vi "MAIN.vi"() -> ()   [LabVIEW 2015]
doc: "Use this template to create an application that executes repeatedly until you click the Stop button. This template polls the state of the Stop button and does not use events. Use the Top-Level Application template (not available in the Base package) to create a single-loop application with event handling."
uses:
  <vilib>/event_ctls.llb/eventvkey.ctl
  <vilib>/Utility/miscctls.llb/LVPointTypeDef.ctl
  SUB_Load and Save Controls.llb/RWC_Actions.ctl
  <vilib>/Utility/miscctls.llb/LVRowAndColumnTypeDef.ctl
  <vilib>/Utility/sysdir.llb/System Directory Type.ctl
  <vilib>/Utility/NIReport.llb/image depth.ctl
  <vilib>/Analysis/baseanly.llb/Mean (DBL).vi
  <vilib>/Utility/config.llb/Read Key (String).vi
  <vilib>/addons/_office/excel.llb/Excel Easy Table (str).vi
  <vilib>/Utility/config.llb/Write Key (String).vi
  <vilib>/Utility/NIReport.llb/NI_report.lvclass
  <vilib>/Utility/config.llb/NI_LVConfig.lvlib
  <vilib>/Analysis/NI_AALBase.lvlib
  <vilib>/addons/_office/NI_ReportGenerationToolkit.lvlib
  <vilib>/Utility/NIReport.llb/NI_ReportGenerationCore.lvlib
  <vilib>/Utility/NIReport.llb/Excel/NI_Excel.lvclass
  <vilib>/Analysis/NI_AALPro.lvlib
panel:
  out "FTS 동작시험 상태":T1="시험 시작"
  out "시험 프로파일":string[][](array[string])=[["Init(1)-35lb", "35", "5000"], ["Init(2)-70lb", "70", "5000"], ["Load(1)-0lb", "0", "3000"], ["Load(2)-5lb", "5", "3000"], ["Load(3)-10lb", "10", "3000"], ["Load(4)-20lb", "20", "3000"], ["Load(5)-30lb", "30", "3000"], ["Load(6)-40lb", "40", "3000"]]
  in  "필터 업데이트":bool
  out "CDC 평균 카운터":i32=10
  out "log refnum":refnum<file> caption="참조 번호 복제"
  out "ms 타이머 값":u32=14257885
  out "Logging No.":u32
  in  "Data Logging":bool caption="Data Logging (Desktop folder)"
  in  "CDC-평균데이터 처리 완료":bool
  out "CDC Averagedata":T2 caption="CDC Average data" {"Right Wing-C, C6/C0" format="%#.9f"; "Right Wing-B, C5/C0" format="%#.9f"; "Right Wing-A, C4/C0" format="%#.9f"; "Left Wing-C, C3/C0" format="%#.9f"; "Left Wing-B, C2/C0" format="%#.9f"; "Left Wing-A, C1/C0" format="%#.9f"}
  in  "평균데이터 취득-CDC":bool
  out "CDC 평균 버퍼":cluster{"Count":i32, "CDC Data Buffer":T2[]} {"CDC Data Buffer"."Right Wing-C, C6/C0" format="%#.9f"; "CDC Data Buffer"."Right Wing-B, C5/C0" format="%#.9f"; "CDC Data Buffer"."Right Wing-A, C4/C0" format="%#.9f"; "CDC Data Buffer"."Left Wing-C, C3/C0" format="%#.9f"; "CDC Data Buffer"."Left Wing-B, C2/C0" format="%#.9f"; "CDC Data Buffer"."Left Wing-A, C1/C0" format="%#.9f"}
  out "RxD":string
  out "그래프 타이머 값 2":u32=14257934
  out "창크게":bool
  out "통신에러카운트 1":i32
  out "그래프 타이머 값 1":u32=14257934
  in  "설정값 불러오기":bool=TRUE
  out "ACT-RS232":bool
  in  "보드 통신 연결 1":bool
  in  "포트닫기 1":bool
  in  "포트오픈 1":bool
  in  "탭-Top":T3(tab)=enum."Utilty"
  in  "Filter Enable (CDC)":bool
  out "CDC Status":u32=65536 format="%06x"
  out "CDC Offet":T2 caption="CDC Offset data" {"Right Wing-C, C6/C0" format="%#.9f"; "Right Wing-B, C5/C0" format="%#.9f"; "Right Wing-A, C4/C0" format="%#.9f"; "Left Wing-C, C3/C0" format="%#.9f"; "Left Wing-B, C2/C0" format="%#.9f"; "Left Wing-A, C1/C0" format="%#.9f"}
  in  "그래프 반출 1":bool
  in  "그래프 지우기 1":bool
  out "CDC(PCAP02) Graph":waveform(dbl)[](graph)=[{"t0"=timestamp(3554680480.5032296 s since 1904-01-01), "dt"=0.10200000000000001, "Y"=[0.9929709434509277]}, {"t0"=timestamp(3554680480.5032296 s since 1904-01-01), "dt"=0.10200000000000001, "Y"=[0.9975447654724121]}, {"t0"=timestamp(3554680480.5032296 s since 1904-01-01), "dt"=0.10200000000000001, "Y"=[0.9987750053405762]}, {"t0"=timestamp(3554680480.5032296 s since 1904-01-01), "dt"=0.10200000000000001, "Y"=[1.0097055435180664]}, {"t0"=timestamp(3554680480.5032296 s since 1904-01-01), "dt"=0.10200000000000001, "Y"=[1.0132465362548828]}, {"t0"=timestamp(3554680480.5032296 s since 1904-01-01), "dt"=0.10200000000000001, "Y"=[1.0090084075927734]}]
  out "CDC data":T2 caption="CDC Monitoring data" {"Right Wing-C, C6/C0" format="%#.9f"; "Right Wing-B, C5/C0" format="%#.9f"; "Right Wing-A, C4/C0" format="%#.9f"; "Left Wing-C, C3/C0" format="%#.9f"; "Left Wing-B, C2/C0" format="%#.9f"; "Left Wing-A, C1/C0" format="%#.9f"}
  in  "Offset 1":bool
  in  "Filter Enable (IMU)":bool
  out "IMU Offet":T4 caption="IMU Offset data" {"Accelerometer Z" format="%#.9f"; "Accelerometer Y" format="%#.9f"; "Accelerometer X" format="%#.9f"; "Gyroscope Z" format="%#.9f"; "Gyroscope Y" format="%#.9f"; "Gyroscope X" format="%#.9f"}
  out "IMU Graph":waveform(dbl)[](graph)=[{"t0"=timestamp(3554680480.5032296 s since 1904-01-01), "dt"=0.10200000000000001, "Y"=[3.465625]}, {"t0"=timestamp(3554680480.5032296 s since 1904-01-01), "dt"=0.10200000000000001, "Y"=[-2.45625]}, {"t0"=timestamp(3554680480.5032296 s since 1904-01-01), "dt"=0.10200000000000001, "Y"=[-1.45875]}, {"t0"=timestamp(3554680480.5032296 s since 1904-01-01), "dt"=0.10200000000000001, "Y"=[-0.014274]}, {"t0"=timestamp(3554680480.5032296 s since 1904-01-01), "dt"=0.10200000000000001, "Y"=[0.000305]}, {"t0"=timestamp(3554680480.5032296 s since 1904-01-01), "dt"=0.10200000000000001, "Y"=[1.025959]}]
  in  "그래프 지우기 2":bool
  in  "그래프 반출 2":bool
  out "IMU data":T4 caption="IMU Monitoring data" {"Accelerometer Z" format="%#.9f"; "Accelerometer Y" format="%#.9f"; "Accelerometer X" format="%#.9f"; "Gyroscope Z" format="%#.9f"; "Gyroscope Y" format="%#.9f"; "Gyroscope X" format="%#.9f"}
  in  "Offset 2":bool
  in  "Load(lb)":dbl=10.0 min=0.0 max=150.0 step=0.1
  in  "Test name":string="Noname"
  out "Load vs Ratio Graph":cluster{dbl[], dbl[]}[](graph)
  in  "Mark10 Gauge (lb)":dbl format="%.2f"
  out "Test Status":string
  out "Test Data table":string[][](table)=[["-", "-", "-", "-", "-", "-", "-", "-", "-", "-"], ["-", "-", "-", "-", "-", "-", "-", "-", "-", "-"], ["-", "-", "-", "-", "-", "-", "-", "-", "-", "-"], ["-", "-", "-", "-", "-", "-", "-", "-", "-", "-"], ["-", "-", "-", "-", "-", "-", "-", "-", "-", "-"], ["-", "-", "-", "-", "-", "-", "-", "-", "-", "-"], ["-", "-", "-", "-", "-", "-", "-", "-", "-", "-"], ["-", "-", "-", "-", "-", "-", "-", "-", "-", "-"], ["-", "-", "-", "-", "-", "-", "-", "-", "-", "-"]]
  in  "Test Start":bool
  in  "Port-FTS":refnum<visa-resource-name>="COM5" caption="FTS \nCOM port"
  in  "FTS Testing":bool
  out "FTS comm.":bool
  in  "Force Set":bool
  in  "Filter Simul":bool
  in  "Response Time":bool
  in  "Noise level Analysis":bool
  in  "Fitting Coefficient":string="\tLeft Wing-A\tLeft Wing-B\tLeft Wing-C\tRight Wing-A\tRight Wing-B\tRight Wing-C\n Coefficient X^0\t0.048738964\t0.151323172\t0.20577303\t0.048738964\t0.151323172\t0.20577303\nCoefficient X^1\t44014.76964\t56340.67608\t56151.02084\t44014.76964\t56340.67608\t56151.02084\nCoefficient X^2\t9601377.151\t-117410867.8\t-91851520.34\t9601377.151\t-117410867.8\t-91851520.34\nCoefficient X^3\t-37149802732\t3.36742E+11\t1.45413E+11\t-37149802732\t3.36742E+11\t1.45413E+11\n"
  out "CDC data(lb)":T2 caption="CDC  data (lb)" {"Right Wing-C, C6/C0" format="%#.9f"; "Right Wing-B, C5/C0" format="%#.9f"; "Right Wing-A, C4/C0" format="%#.9f"; "Left Wing-C, C3/C0" format="%#.9f"; "Left Wing-B, C2/C0" format="%#.9f"; "Left Wing-A, C1/C0" format="%#.9f"}
  out "수신 실패(T) 1":bool=TRUE
  out "보드-통신상태 1":bool caption="Status"
  out "*Board ID1":string="None...." caption="F/W Ver."
  in  "Port-set 1":refnum<visa-resource-name>="COM4" caption="COM port"
  out "Port-act 1":refnum<visa-resource-name>="COM4"
  in  "stop":bool=TRUE
  out "데이터 송수신":bool
  in  "설정값 로드":bool
  out "status string":string="Ready (available after the communication connection)"
  # "GEN4 1st PP - GUI Program"
  # "Ver. 160822A"
  # "Comm. Connection"
  # "115200bps"
  # "Click to delete a offset data"
  # "Gyroscope X"
  # "Gyroscope Y"
  # "Gyro. (dps)"
  # "Gyroscope Z"
  # "Accelerometer X"
  # "Accelerometer Y"
  # "Acc. (g)"
  # "Accelerometer Z"
  # "Click to delete a offset data"
  # "ESM301: 115200bps\nMARK10: 9600bps"
  # "<Response test>"
  # "* Development Tool"
  # "CDC Calibration"
  # "Analysis Tool"
  # "Reserved"
  # "[Monitoring - CDC]\nCDC Monitoring data\n(w/ CDC Offset data)\n\n             ***\n \n[Configuration]\nFitting Coefficient"
  # "<Fitting>\nratio to lb"
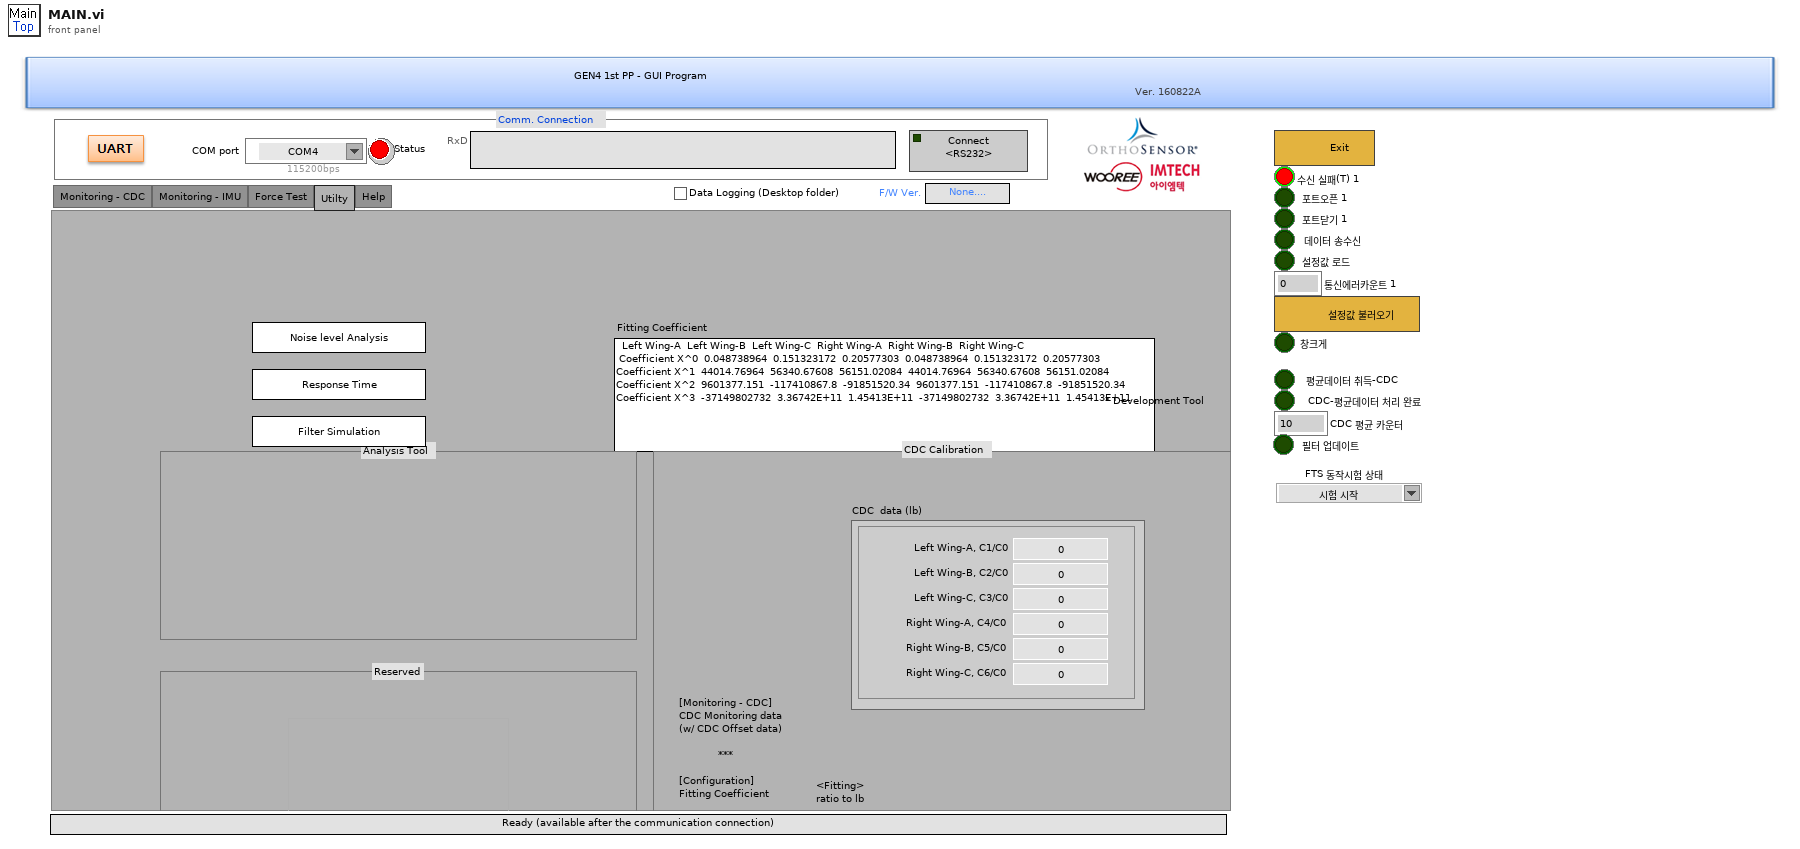
[diagram p1: front panel]
types:
  T1 = typedef "컨트롤-동작시험상태 FTS.ctl" = string
  T2 = typedef "컨트롤-CDC data.ctl" = cluster{"Left Wing-A, C1/C0":dbl, "Left Wing-B, C2/C0":dbl, "Left Wing-C, C3/C0":dbl, "Right Wing-A, C4/C0":dbl, "Right Wing-B, C5/C0":dbl, "Right Wing-C, C6/C0":dbl}
  T3 = enum32{"Monitoring - CDC", "Monitoring - IMU", "Force Test", "Utilty", "Help"}
  T4 = typedef "컨트롤-IMU data.ctl" = cluster{"Gyroscope X":dbl, "Gyroscope Y":dbl, "Gyroscope Z":dbl, "Accelerometer X":dbl, "Accelerometer Y":dbl, "Accelerometer Z":dbl}
  T5 = typedef "컨트롤-동작상태 FTS.ctl" = string
  T6 = typedef "eventvkey.ctl" = enum16{"ASCII", "Enter", "Return", "Shift", "Ctrl", "Alt", "Cmd", "Opt", "Caps", "NumLock", "Clear", "Break", "Up", "Down", "Left", "Right", "Insert", "Delete", "Home", "End", "PageUp", "PageDown", "Escape", "Help", "Pause", "ScrollLock", "F1", "F2", "F3", "F4", "F5", "F6", "F7", "F8", "F9", "F10", "F11", "F12", "F13", "F14", "F15", "F16", "F17", "F18", "F19", "F20", "F21", "F22", "F23", "F24", "Play", "VolumeUp", "VolumeDown", "Mute", "Two Byte Char"}
  T7 = typedef "RWC_Actions.ctl" = enum16{"Read", "Write", "Read and Create"}
  T8 = enum16{"Always On", "Always Off", "Off While Running"}
  T9 = typedef "LVPointTypeDef.ctl" = cluster{"Horizontal":i16, "Vertical":i16}
  T10 = typedef "LVRowAndColumnTypeDef.ctl" = cluster{"Row":i32, "Column":i32}
  T11 = enum16{"open", "replace", "create", "open or create", "replace or create", "replace or create with confirmation"}
  T12 = cluster{"position (Excel)":cluster{"row":i32, "column":i32}, "name (Excel)":string, "bookmark (Word)":string}
  T13 = enum16{"Standard Report", "HTML", "Word", "Excel"}
  T14 = enum16{"maximized", "minimized", "normal", "no change"}
  T15 = typedef "컨트롤-설정값 선택.ctl" = string
  T16 = typedef "NI_LVConfig.lvlib/Config Data RefNum.ctl" = refnum<k1>
  T17 = typedef "System Directory Type.ctl" = i32
  T18 = typedef "NI_ReportGenerationCore.lvlib/image depth.ctl" = u16
  T19 = typedef "LVRectTypeDef.ctl" = cluster{"Left":i16, "Top":i16, "Right":i16, "Bottom":i16}
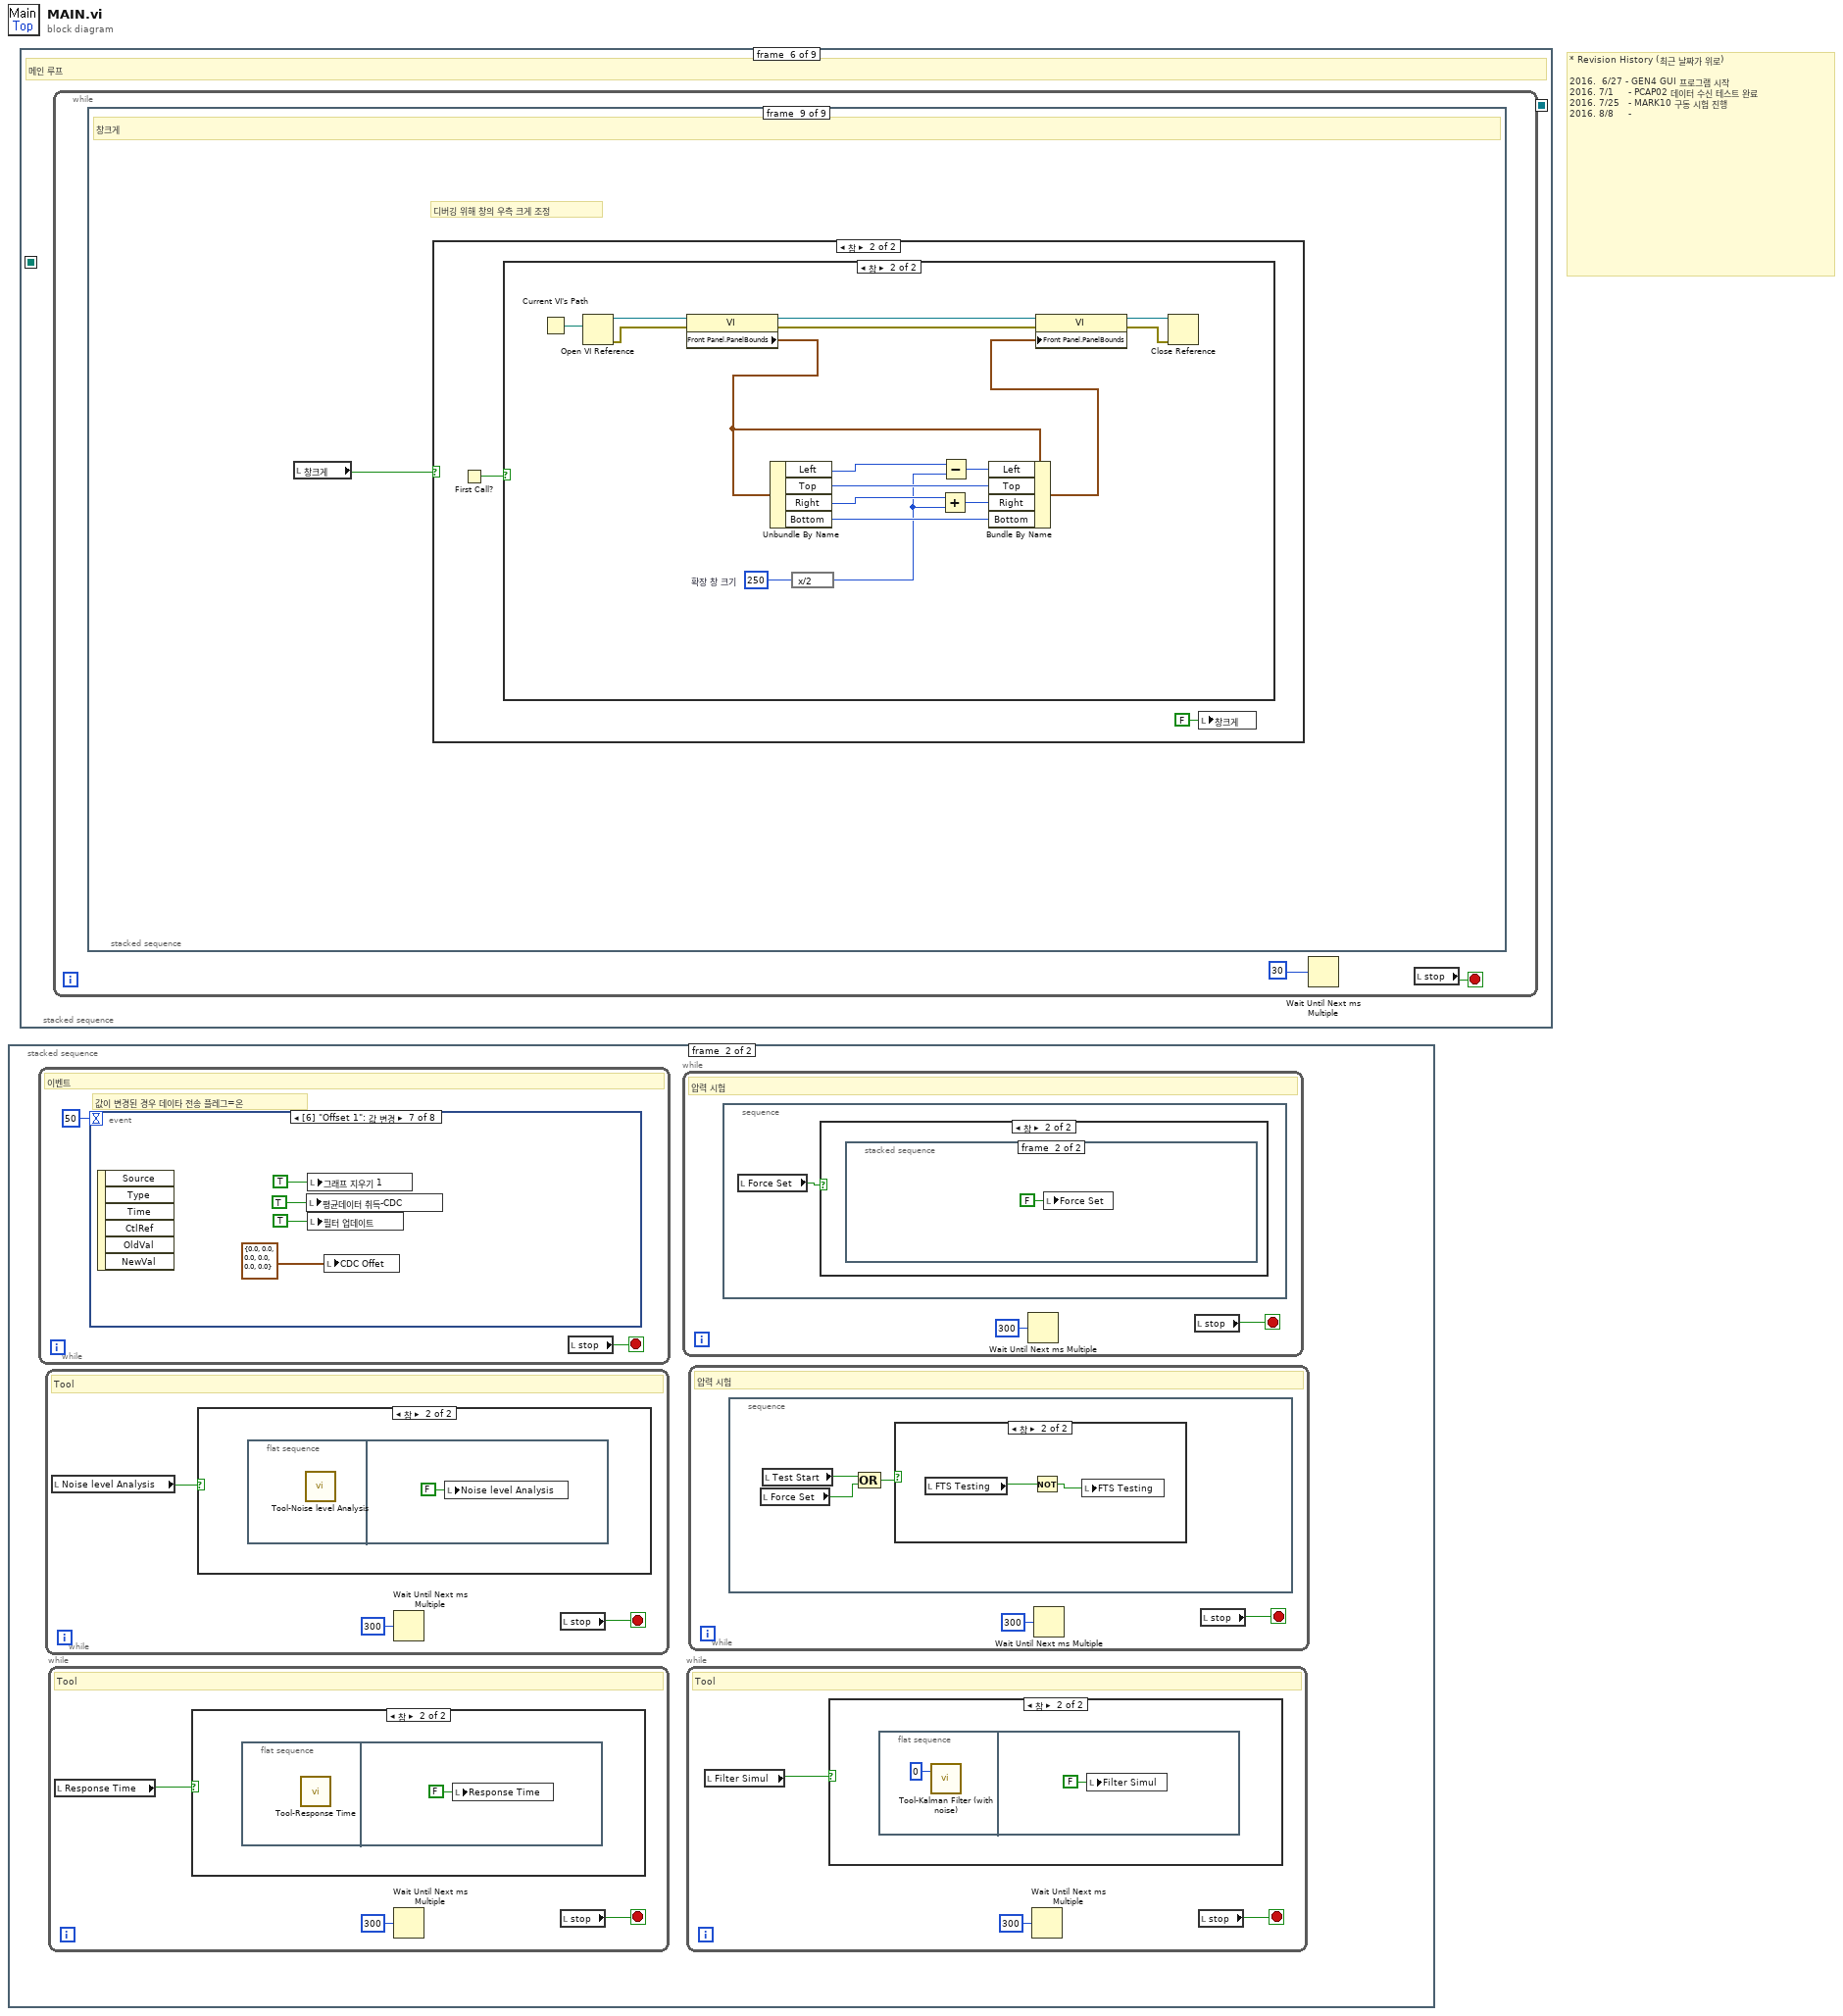
[diagram p0: block diagram]
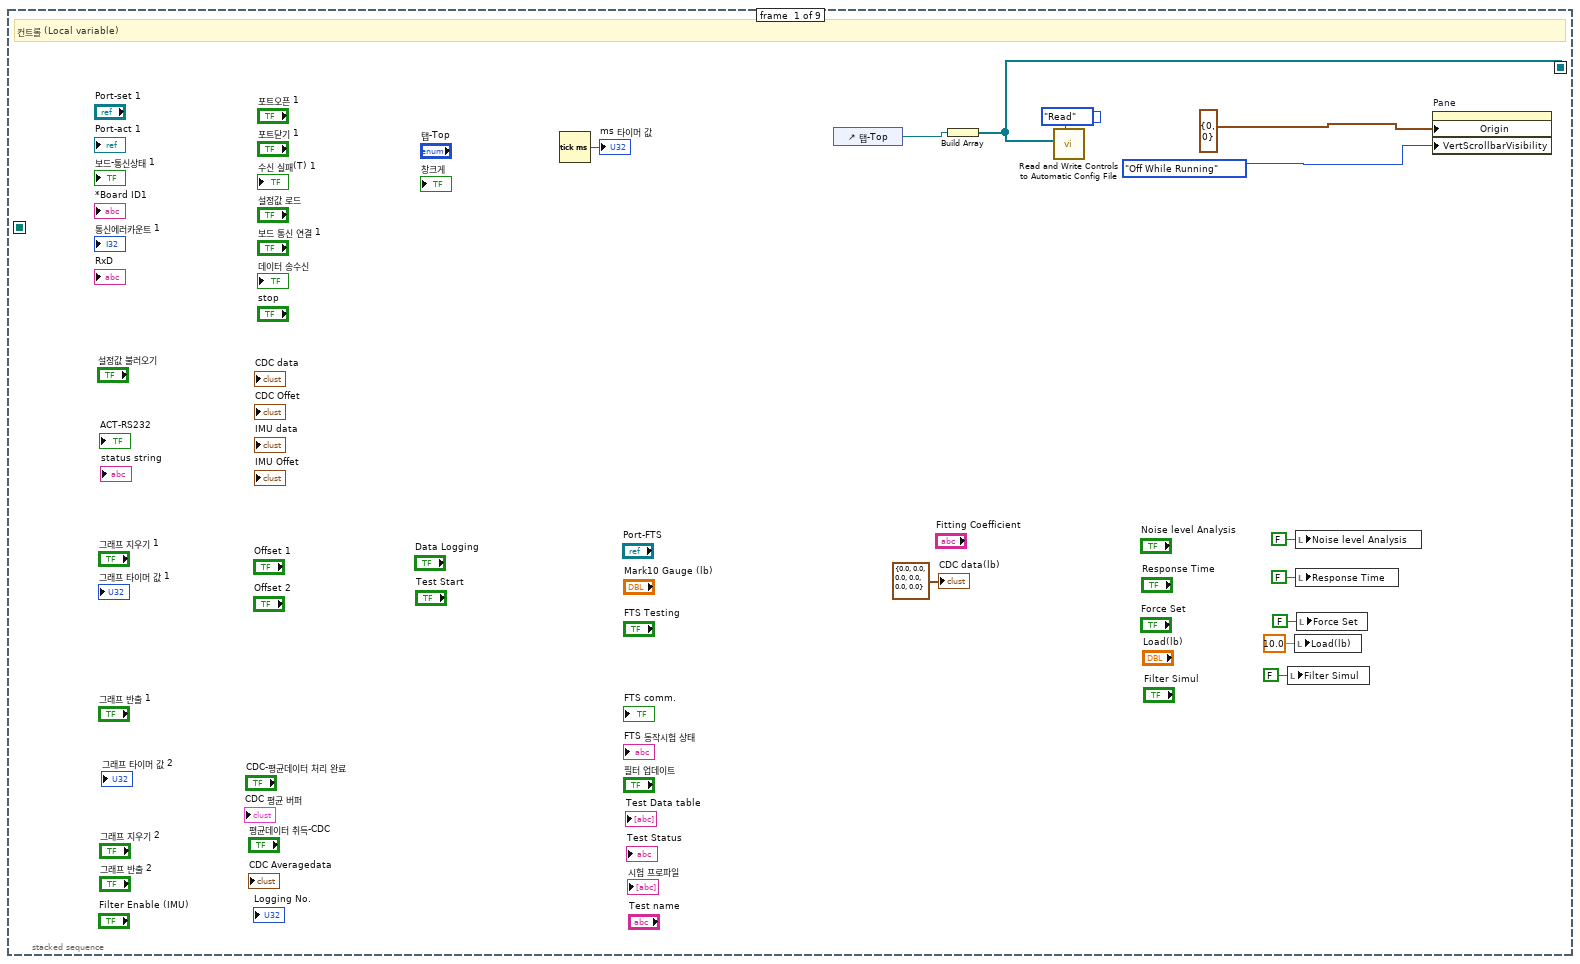
[diagram p2: hidden frame]
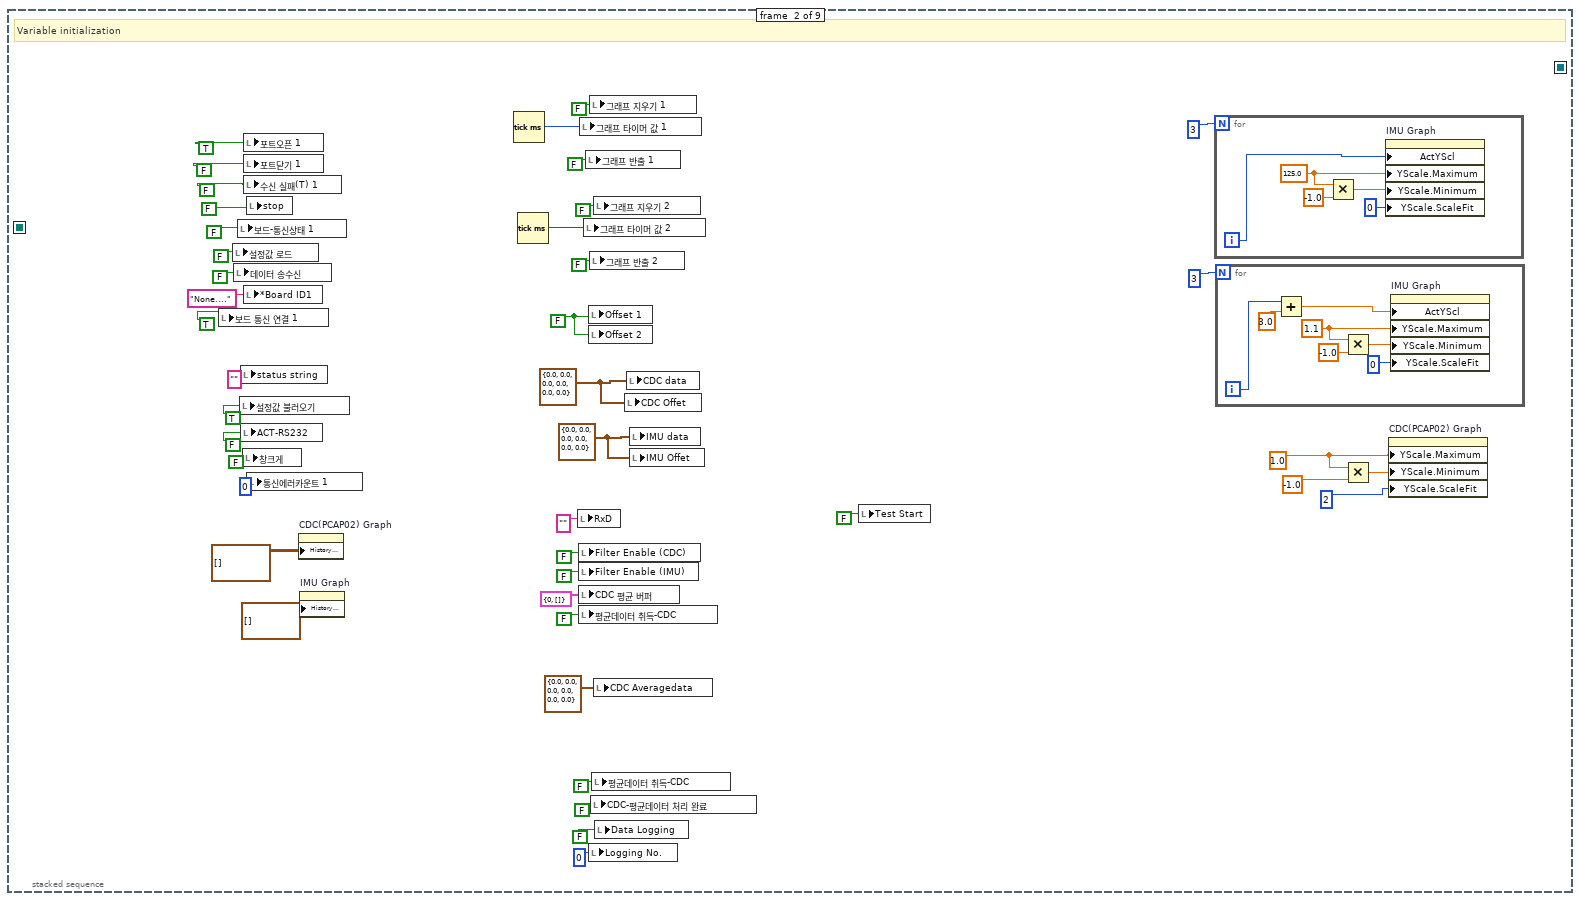
[diagram p3: hidden frame]
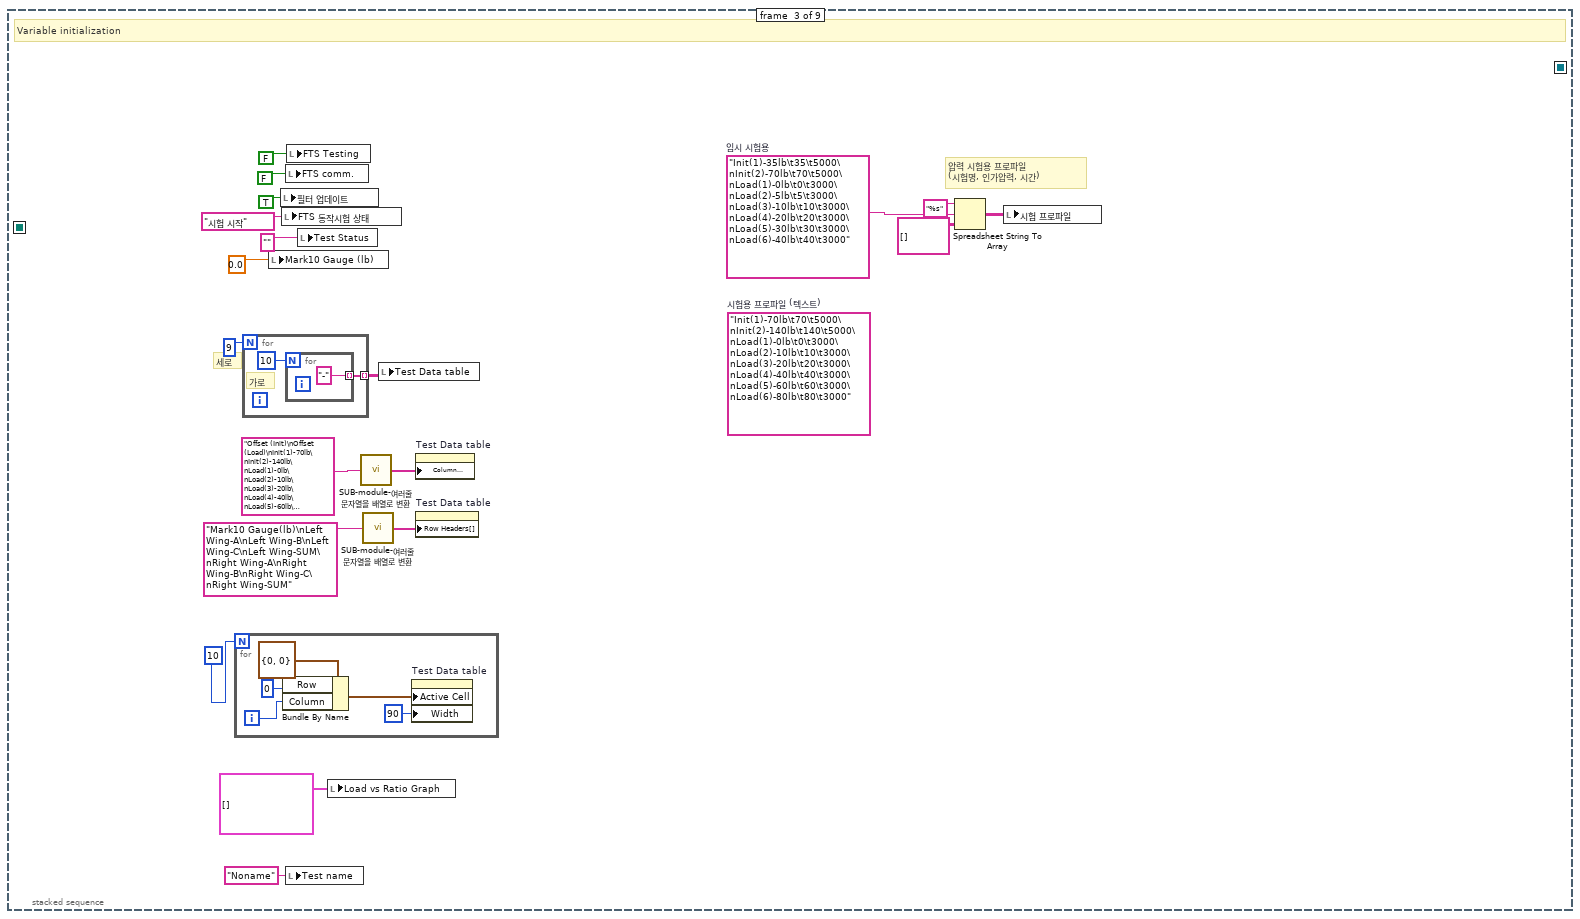
[diagram p4: hidden frame]
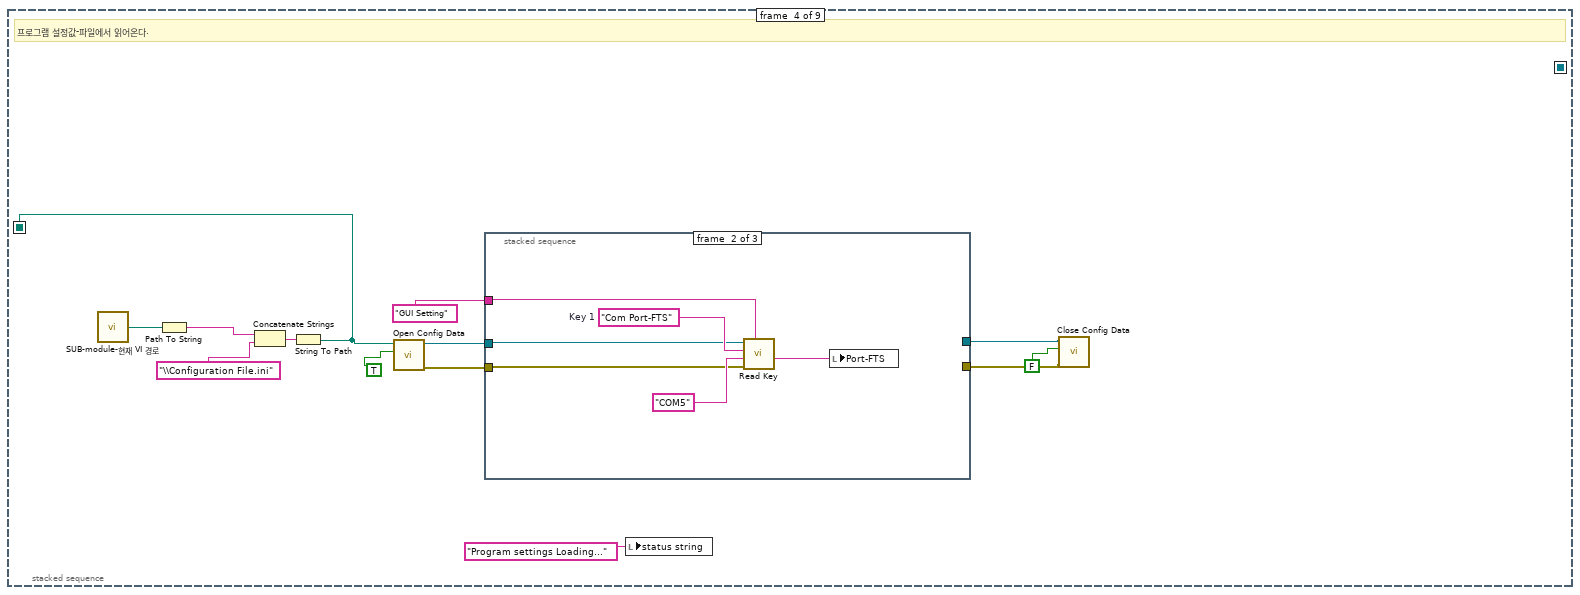
[diagram p5: hidden frame]
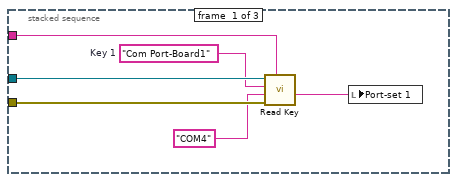
[diagram p6: hidden frame]
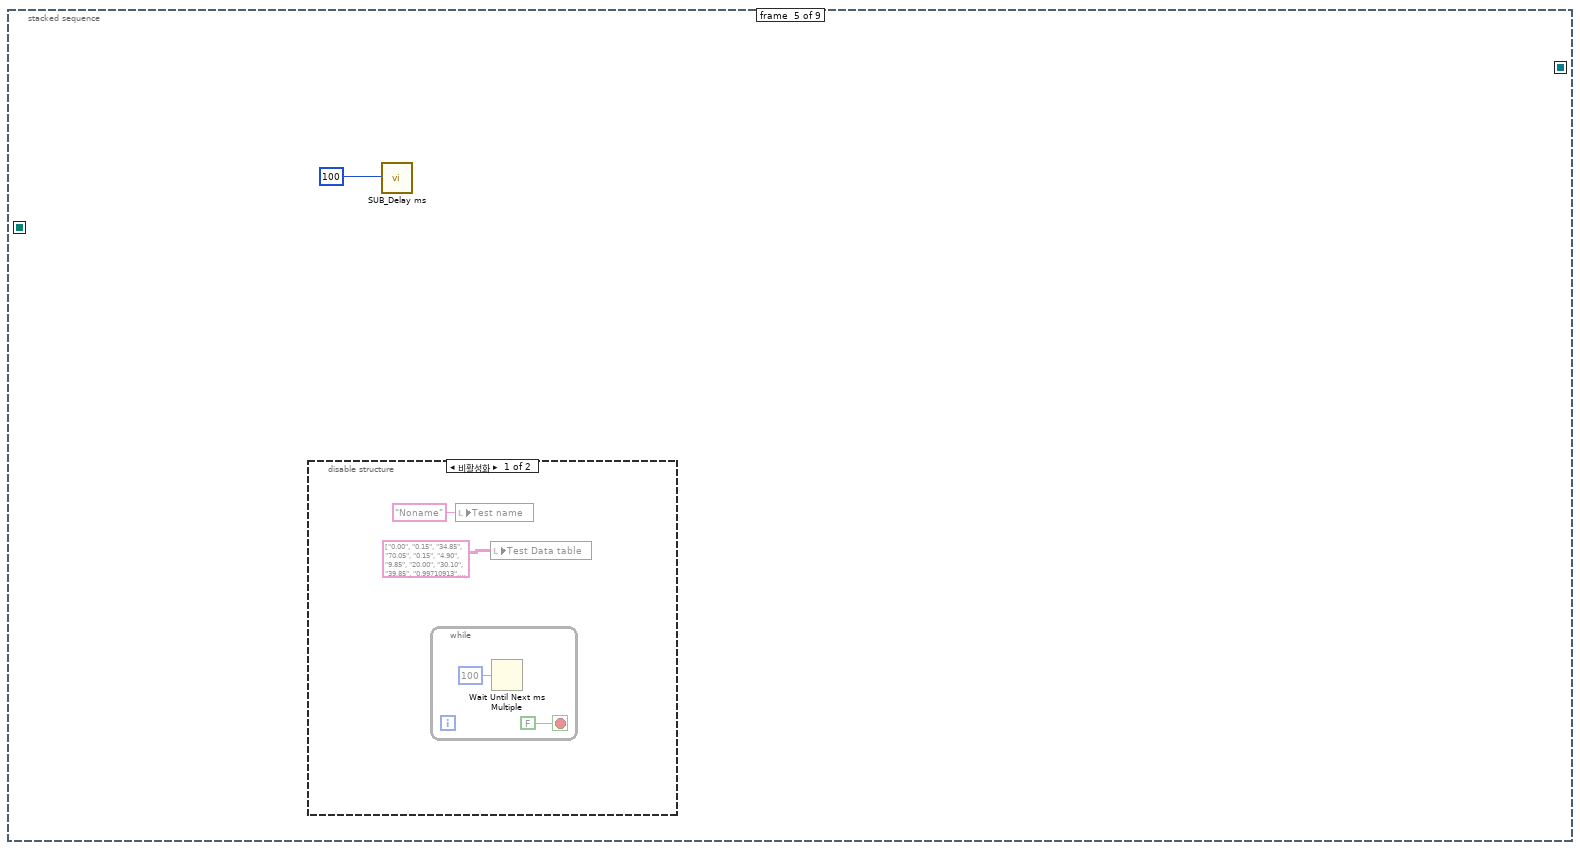
[diagram p8: hidden frame]
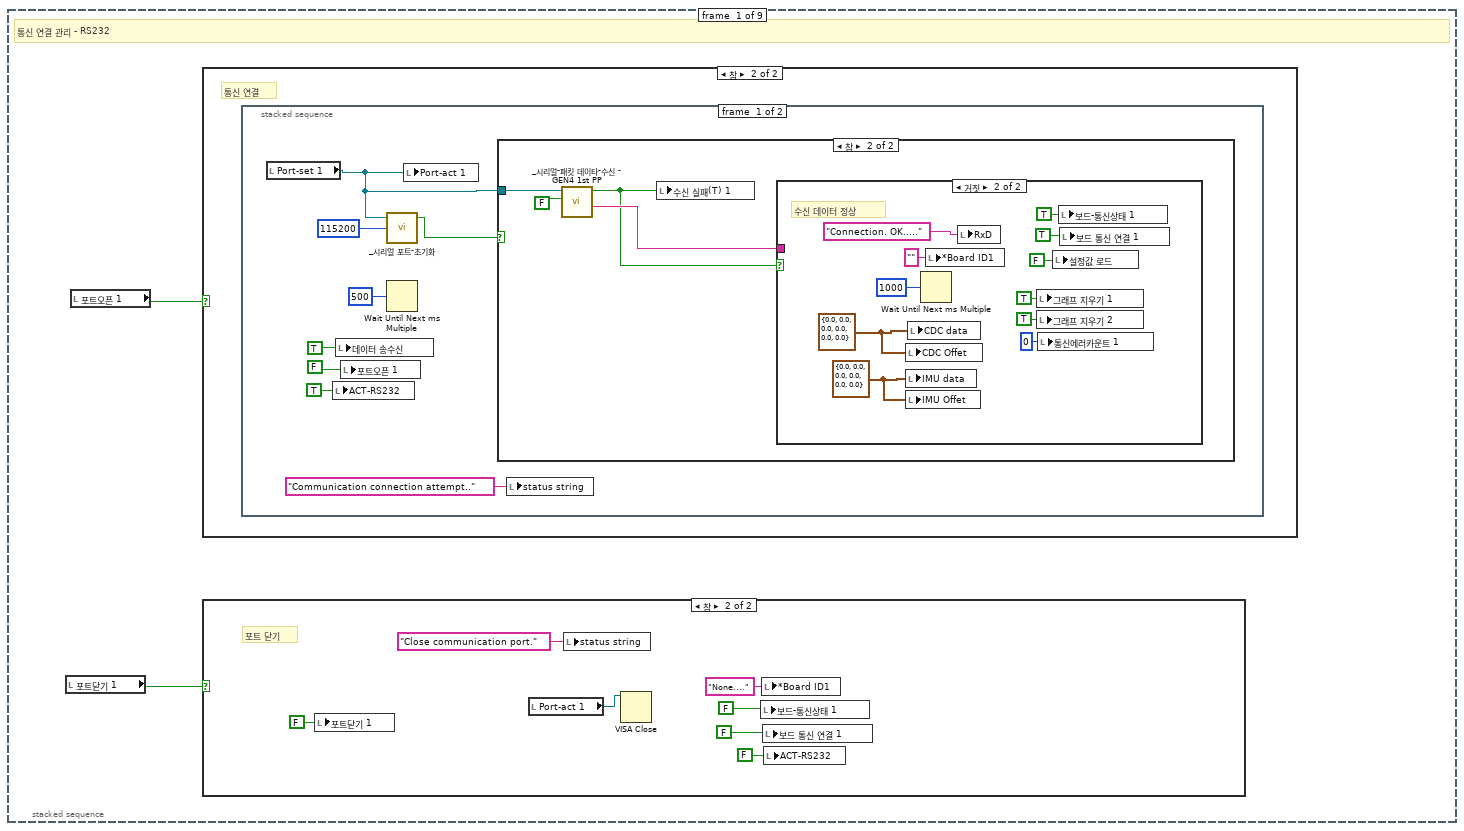
[diagram p10: hidden frame]
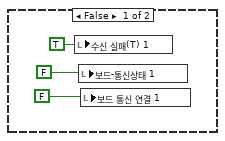
[diagram p12: hidden frame]
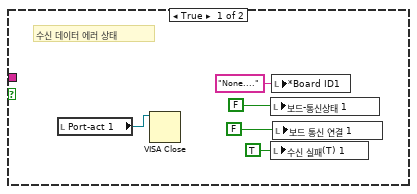
[diagram p13: hidden frame]
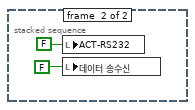
[diagram p14: hidden frame]
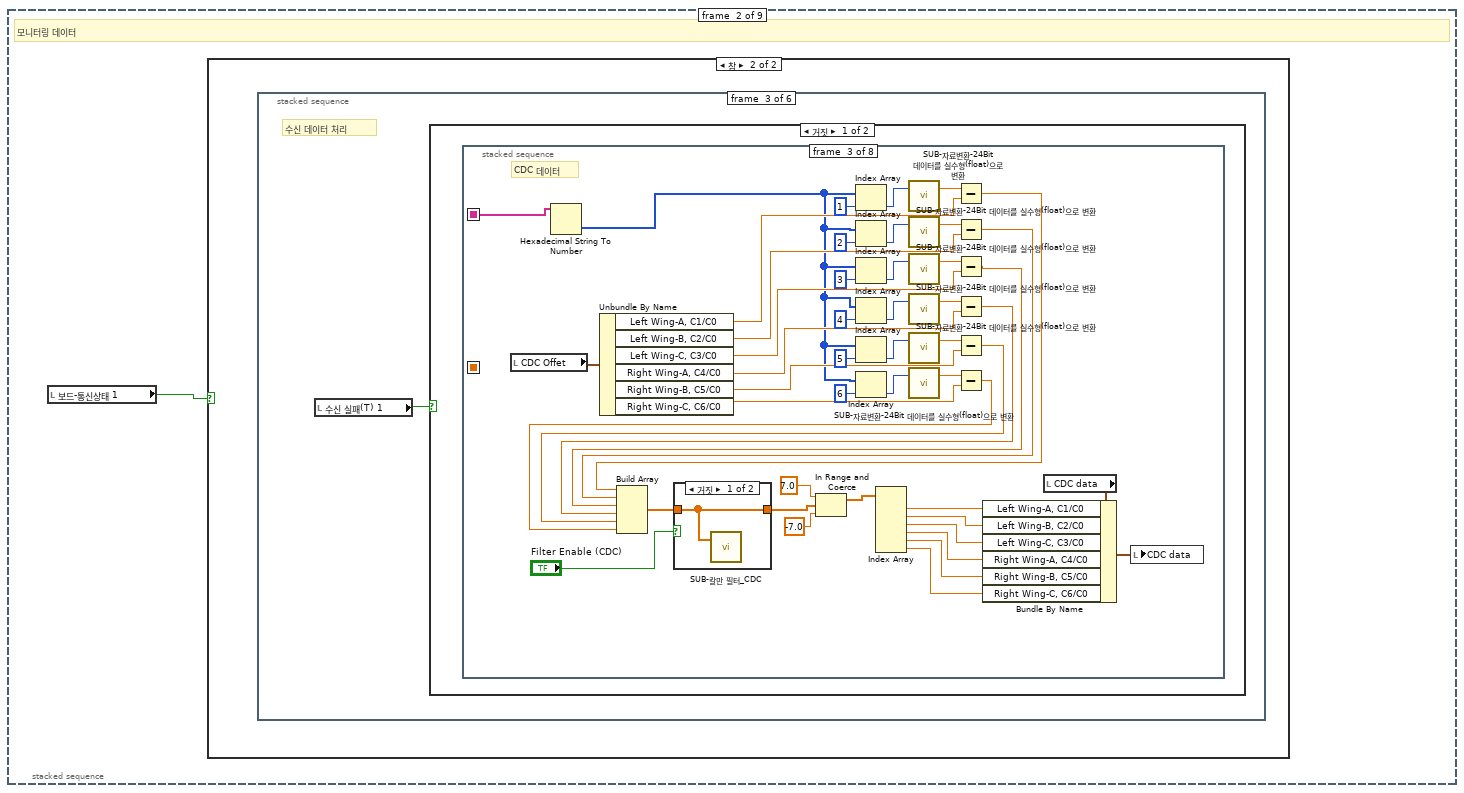
[diagram p16: hidden frame]
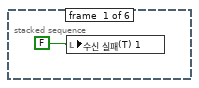
[diagram p18: hidden frame]
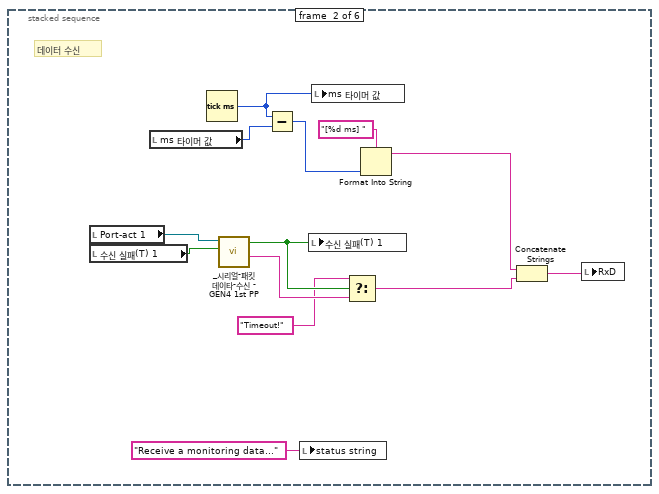
[diagram p19: hidden frame]
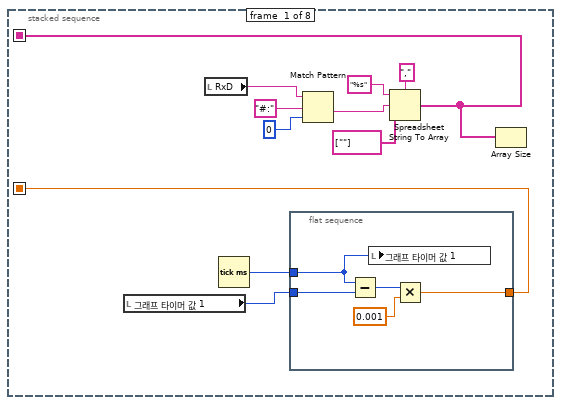
[diagram p20: hidden frame]
diagram:
  # "* Revision History (최근 날짜가 위로)\n\n2016.  6/27 - GEN4 GUI 프로그램 시작\n2016. 7/1     - PCAP02 데이터 수신 테스트 완료\n2016. 7/25   - MARK10 구동 시험 진행\n2016. 8/8     -"
  n1 = stacked-sequence {
    frame #0 {
      n2 = call "SUB_Delay ms.vi"("delay(ms)"=u32 300) -> ()  [unwired: 3 in]
    }
    frame #1 {
      n3 = while {
        stop <- w33 stop-if-true
        # "값이 변경된 경우 데이타 전송 플레그=온"
        # "이벤트"
        n4 = event shown="[6] \"Offset 1\": 값 변경" {
          selector: _ -> [_ _ _ _ _ _ _ _]
          dyn-events: _ -> [_ _ _ _ _ _ _ _]
          timeout: 50 -> [_ _ _ _ _ _ _ _]
          event Timeout {
            n5 = event-data() -> ()  [unwired: 3 out]
          }
          event Key Down {
            # "Ctrl + 1"
            n6 = event-data() -> ("Char"=w41:i16, "VKey"=w39:T6, "Mods"=w43:cluster{"Num Pad":bool, "Menu Key":bool})  [unwired: 6 out]
            n7 = Unbundle By Name(w43) -> ("Menu Key"=w35:bool)
            n8 = Equal?(x=eventvkey."ASCII" ("V 키"), y=w39) -> (x = y?=w37:bool)
            n9 = Equal?(x=i16 49 ("문자"), y=w41) -> (x = y?=w38:bool)
            n10 = And(x=w38, y=w37) -> (x .and. y?=w36:bool)
            n11 = And(x=w36, y=w35) -> (x .and. y?=w34:bool)
            n12 = case shown="참" w34 {
              frame False {
              }
              frame True {
                n13 = local write "창크게"(TRUE ("창크게")) -> ()
              }
            }
          }
          event "보드 통신 연결 1": Value Change {
            n14 = event-data() -> ("NewVal"=w45:bool)  [unwired: 6 out]
            n15 = case shown="참" w45 {
              frame False {
                # "통신 닫기"
                n16 = local write "포트오픈 1"(FALSE) -> ()
                n17 = local write "포트닫기 1"(TRUE) -> ()
              }
              frame True {
                # "통신 연결"
                n18 = local write "포트오픈 1"(TRUE) -> ()
                n19 = local write "포트닫기 1"(FALSE) -> ()
              }
            }
          }
          event "설정값 불러오기": Value Change {
            n20 = event-data() -> ("NewVal"=w50:bool)  [unwired: 6 out]
            n21 = case shown="참" w50 {
              frame False {
              }
              frame True {
                n22 = local write "설정값 로드"(TRUE ("Power On Flag")) -> ()
              }
            }
          }
          event Mouse Down? {
            n23 = event-data() -> ()  [unwired: 9 out]
            n24 = local write "필터 업데이트"(TRUE ("필터 업데이트")) -> ()
            n25 = local write "그래프 지우기 1"(TRUE ("그래프 지우기")) -> ()
            n26 = local write "CDC Offet"(T2 {"Left Wing-A, C1/C0"=0.0, "Left Wing-B, C2/C0"=0.0, "Left Wing-C, C3/C0"=0.0, "Right Wing-A, C4/C0"=0.0, "Right Wing-B, C5/C0"=0.0, "Right Wing-C, C6/C0"=0.0} ("CDC data")) -> ()
            n27 = event-data() -> ()  [unwired: 2 in, 1 out]
          }
          event Mouse Down? {
            n28 = event-data() -> ()  [unwired: 9 out]
            n29 = local write "그래프 지우기 2"(TRUE ("그래프 지우기")) -> ()
            n30 = local write "IMU Offet"(T4 {"Gyroscope X"=0.0, "Gyroscope Y"=0.0, "Gyroscope Z"=0.0, "Accelerometer X"=0.0, "Accelerometer Y"=0.0, "Accelerometer Z"=0.0} ("IMU data")) -> ()
            n31 = event-data() -> ()  [unwired: 2 in, 1 out]
          }
          event "Offset 1": Value Change {
            n32 = event-data() -> ()  [unwired: 7 out]
            n33 = local write "평균데이터 취득-CDC"(TRUE ("CDC-평균데이터 처리 완료")) -> ()
            n34 = local write "그래프 지우기 1"(TRUE ("그래프 지우기")) -> ()
            n35 = local write "필터 업데이트"(TRUE ("필터 업데이트")) -> ()
            n36 = local write "CDC Offet"(T2 {"Left Wing-A, C1/C0"=0.0, "Left Wing-B, C2/C0"=0.0, "Left Wing-C, C3/C0"=0.0, "Right Wing-A, C4/C0"=0.0, "Right Wing-B, C5/C0"=0.0, "Right Wing-C, C6/C0"=0.0} ("CDC data")) -> ()
          }
          event Panel Close? {
            n37 = event-data() -> ()  [unwired: 5 out]
            n38 = local write "stop"(TRUE ("stop")) -> ()
            n39 = event-data("Discard?"=TRUE ("stop")) -> ()  [unwired: 1 in, 1 out]
          }
        }
        n40 = local read "stop"() -> (w33:bool)
      }
      n41 = while {
        stop <- w12 stop-if-true
        # "Tool"
        n42 = local read "Noise level Analysis"() -> (w11:bool)
        n43 = case shown="참" w11 {
          frame False {
          }
          frame True {
            n44 = flat-sequence {
              frame #0 {
                n45 = call "Tool-Noise level Analysis.vi"() -> ()  [unwired: 6 in]
              }
              frame #1 {
                n46 = local write "Noise level Analysis"(FALSE ("Noise level Analysis")) -> ()
              }
            }
          }
        }
        n47 = Wait Until Next ms Multiple(millisecond multiple=u32 300 ("ms 배수")) -> ()  [unwired: 1 out]
        n48 = local read "stop"() -> (w12:bool)
      }
      n49 = while {
        stop <- w8 stop-if-true
        # "Tool"
        n50 = local read "Response Time"() -> (w7:bool)
        n51 = case shown="참" w7 {
          frame False {
          }
          frame True {
            n52 = flat-sequence {
              frame #0 {
                n53 = call "Tool-Response Time.vi"() -> ()  [unwired: 4 in]
              }
              frame #1 {
                n54 = local write "Response Time"(FALSE ("Response Time")) -> ()
              }
            }
          }
        }
        n55 = Wait Until Next ms Multiple(millisecond multiple=u32 300 ("ms 배수")) -> ()  [unwired: 1 out]
        n56 = local read "stop"() -> (w8:bool)
      }
      n57 = while {
        stop <- w23 stop-if-true
        # "압력 시험"
        n58 = stacked-sequence {
          frame #0 {
            n59 = local read "Force Set"() -> (w25:bool)
            n60 = case shown="참" w25 {
              frame False {
              }
              frame True {
                n61 = stacked-sequence {
                  frame #0 {
                    n62 = local read "Port-FTS"() -> (w29:refnum<visa-resource-name>)
                    n63 = local read "Load(lb)"() -> (w28:dbl)
                    n64 = call "_시리얼_Mark10-제어 (압력설정).vi"("FTS 제어 상태"=T5 "압력제어 시작", "압력 설정(lb)"=w28, "시리얼 포트"=w29) -> ("통신 정상"=w26:bool)  [unwired: 2 out]
                    n65 = case shown="거짓" w26 {
                      frame False {
                        n66 = One Button Dialog(message="Can't find equipment!" ("메시지")) -> ()  [unwired: 1 in, 1 out]
                      }
                      frame True {
                      }
                    }
                  }
                  frame #1 {
                    n67 = local write "Force Set"(FALSE ("Force Set")) -> ()
                  }
                }
              }
            }
          }
        }
        n68 = Wait Until Next ms Multiple(millisecond multiple=u32 300 ("ms 배수")) -> ()  [unwired: 1 out]
        n69 = local read "stop"() -> (w23:bool)
      }
      n70 = while {
        stop <- w3 stop-if-true
        # "Tool"
        n71 = local read "Filter Simul"() -> (w2:bool)
        n72 = case shown="참" w2 {
          frame False {
          }
          frame True {
            n73 = flat-sequence {
              frame #0 {
                n74 = call "Tool-Kalman Filter (with noise).vi"("프런트패널 윈도우:모니터"=u16 0) -> ()  [unwired: 3 in]
              }
              frame #1 {
                n75 = local write "Filter Simul"(FALSE ("Filter Simul")) -> ()
              }
            }
          }
        }
        n76 = Wait Until Next ms Multiple(millisecond multiple=u32 300 ("ms 배수")) -> ()  [unwired: 1 out]
        n77 = local read "stop"() -> (w3:bool)
      }
      n78 = while {
        stop <- w15 stop-if-true
        # "압력 시험"
        n79 = stacked-sequence {
          frame #0 {
            n80 = local read "Force Set"() -> (w18:bool)
            n81 = local read "Test Start"() -> (w19:bool)
            n82 = Compound Arithmetic op=OR ("복합 연산")(w19, w18) -> (w17:bool)
            n83 = case shown="참" w17 {
              frame False {
                n84 = local write "FTS Testing"(FALSE ("FTS 시험 진행")) -> ()
              }
              frame True {
                n85 = local read "FTS Testing"() -> (w22:bool)
                n86 = Not(x=w22) -> (.not. x?=w21:bool)
                n87 = local write "FTS Testing"(w21) -> ()
              }
            }
          }
        }
        n88 = Wait Until Next ms Multiple(millisecond multiple=u32 300 ("ms 배수")) -> ()  [unwired: 1 out]
        n89 = local read "stop"() -> (w15:bool)
      }
    }
  }
  n90 = stacked-sequence {
    seq-local: [_ _ _ w160 _ _ _ _ _] -> [_ _ _ _ _ _ _ w1082 _]
    seq-local: [w72 _ _ _ _ _ _ _ _] -> [_ _ _ _ _ _ _ w1078 _]
    frame #0 {
      # "컨트롤 (Local variable)"
      n91 = Tick Count (ms)() -> (millisecond timer value=→"ms 타이머 값":u32)
      n92 = control-ref of="탭-Top"() -> (w70:refnum<vi>)
      n93 = Build Array(w70) -> (w72:refnum<vi>[])
      n94 = call "Read and Write Controls to Automatic Config File.vi"("Action"=RWC_Actions."Read", "Control References"=w72) -> ()  [unwired: 9 in, 1 out]
      n95 = local write "Filter Simul"(FALSE ("Filter Simul")) -> ()
      n96 = local write "Load(lb)"(10.0 ("Load(lb)")) -> ()
      n97 = local write "Noise level Analysis"(FALSE ("Noise level Analysis")) -> ()
      n98 = local write "Response Time"(FALSE ("Response Time")) -> ()
      n99 = local write "Force Set"(FALSE ("Force Set")) -> ()
      n100 = property on="Pane" class="Pane"("Origin"=T9 {"Horizontal"=0, "Vertical"=0} ("원점"), "VertScrollbarVisibility"=T8."Off While Running" ("수직 스크롤 막대 보이기")) -> ()  [unwired: 2 in, 2 out]
      "CDC data(lb)" <- T2 {"Left Wing-A, C1/C0"=0.0, "Left Wing-B, C2/C0"=0.0, "Left Wing-C, C3/C0"=0.0, "Right Wing-A, C4/C0"=0.0, "Right Wing-B, C5/C0"=0.0, "Right Wing-C, C6/C0"=0.0} ("CDC data 2")
    }
    frame #1 {
      w80 = 1.0 ("Y 스케일.범위:최대값")
      w93 = T4 {"Gyroscope X"=0.0, "Gyroscope Y"=0.0, "Gyroscope Z"=0.0, "Accelerometer X"=0.0, "Accelerometer Y"=0.0, "Accelerometer Z"=0.0} ("IMU data")
      w94 = T2 {"Left Wing-A, C1/C0"=0.0, "Left Wing-B, C2/C0"=0.0, "Left Wing-C, C3/C0"=0.0, "Right Wing-A, C4/C0"=0.0, "Right Wing-B, C5/C0"=0.0, "Right Wing-C, C6/C0"=0.0} ("CDC data")
      w95 = FALSE ("Offset 1")
      # "Variable initialization"
      n101 = local write "보드 통신 연결 1"(TRUE ("포트 연결")) -> ()
      n102 = local write "설정값 로드"(FALSE ("Power On Flag")) -> ()
      n103 = local write "데이터 송수신"(FALSE ("Rx")) -> ()
      n104 = local write "보드-통신상태 1"(FALSE ("Connected")) -> ()
      n105 = local write "설정값 불러오기"(TRUE ("설정값 불러오기")) -> ()
      n106 = local write "status string"("" ("status string")) -> ()
      n107 = local write "ACT-RS232"(FALSE ("ACT-RS422")) -> ()
      n108 = local write "창크게"(FALSE ("창크게")) -> ()
      n109 = local write "포트오픈 1"(TRUE) -> ()
      n110 = local write "포트닫기 1"(FALSE) -> ()
      n111 = local write "수신 실패(T) 1"(FALSE) -> ()
      n112 = local write "*Board ID1"("None...." ("*Board ID")) -> ()
      n113 = local write "stop"(FALSE ("stop")) -> ()
      n114 = local write "통신에러카운트 1"(0 ("통신에러카운트")) -> ()
      n115 = property on="CDC(PCAP02) Graph" class="WFChart (엄격한)"("History Data"=waveform(dbl)[][] [] ("히스토리 데이터")) -> ()  [unwired: 2 in, 2 out]
      n116 = property on="IMU Graph" class="WFChart (엄격한)"("History Data"=waveform(dbl)[][] [] ("히스토리 데이터")) -> ()  [unwired: 2 in, 2 out]
      n117 = Tick Count (ms)() -> (millisecond timer value=w104:u32)
      n118 = Tick Count (ms)() -> (millisecond timer value=w97:u32)
      n119 = local write "RxD"("" ("RxD")) -> ()
      n120 = local write "Filter Enable (CDC)"(FALSE ("Filter Enable (CDC)")) -> ()
      n121 = local write "Filter Enable (IMU)"(FALSE ("Filter Enable (IMU)")) -> ()
      n122 = local write "CDC 평균 버퍼"(cluster{"Count":i32, "CDC Data":T2[]} {"Count"=0, "CDC Data"=[]} ("CDC 평균 버퍼")) -> ()
      n123 = local write "평균데이터 취득-CDC"(FALSE ("평균데이터 취득-CDC")) -> ()
      n124 = local write "그래프 타이머 값 1"(w104) -> ()
      n125 = local write "그래프 타이머 값 2"(w97) -> ()
      n126 = local write "그래프 반출 1"(FALSE ("그래프 반출")) -> ()
      n127 = local write "Offset 1"(w95) -> ()
      n128 = local write "Offset 2"(w95) -> ()
      n129 = local write "Logging No."(u32 0 ("Logging No.")) -> ()
      n130 = local write "그래프 지우기 1"(FALSE ("그래프 지우기")) -> ()
      n131 = local write "그래프 반출 2"(FALSE ("그래프 반출")) -> ()
      n132 = local write "CDC-평균데이터 처리 완료"(FALSE ("CDC-평균데이터 처리 완료")) -> ()
      n133 = local write "평균데이터 취득-CDC"(FALSE ("평균데이터 취득-CDC")) -> ()
      n134 = local write "그래프 지우기 2"(FALSE ("그래프 지우기")) -> ()
      n135 = local write "CDC Averagedata"(T2 {"Left Wing-A, C1/C0"=0.0, "Left Wing-B, C2/C0"=0.0, "Left Wing-C, C3/C0"=0.0, "Right Wing-A, C4/C0"=0.0, "Right Wing-B, C5/C0"=0.0, "Right Wing-C, C6/C0"=0.0} ("CDC data")) -> ()
      n136 = local write "Data Logging"(FALSE ("Data Logging")) -> ()
      n137 = local write "CDC Offet"(w94) -> ()
      n138 = local write "CDC data"(w94) -> ()
      n139 = local write "IMU data"(w93) -> ()
      n140 = local write "IMU Offet"(w93) -> ()
      n141 = local write "Test Start"(FALSE ("Test Start")) -> ()
      n142 = for {
        N: 3 -> [_]
        i -> [w125]
        w126 = 125.0 ("Y 스케일.범위:최대값")
        n143 = Multiply(x=w126, y=-1.0 ("Y 스케일.범위:최대값")) -> (x*y=w128:dbl)
        n144 = property on="IMU Graph" class="WFChart (엄격한)"("ActYScl"=w125, "YScale.Maximum"=w126, "YScale.Minimum"=w128, "YScale.ScaleFit"=u8 0 ("Y 스케일.스케일 맞춤")) -> ()  [unwired: 2 in, 2 out]
      }
      n145 = for {
        N: 3 -> [_]
        i -> [w120]
        w121 = 1.1 ("Y 스케일.범위:최대값")
        n146 = Add(x=w120, y=3.0 ("Y 스케일.범위:최대값")) -> (x+y=w118:dbl)
        n147 = Multiply(x=w121, y=-1.0 ("Y 스케일.범위:최대값")) -> (x*y=w123:dbl)
        n148 = property on="IMU Graph" class="WFChart (엄격한)"("ActYScl"=w118, "YScale.Maximum"=w121, "YScale.Minimum"=w123, "YScale.ScaleFit"=u8 0 ("Y 스케일.스케일 맞춤")) -> ()  [unwired: 2 in, 2 out]
      }
      n149 = Multiply(x=w80, y=-1.0 ("Y 스케일.범위:최대값")) -> (x*y=w79:dbl)
      n150 = property on="CDC(PCAP02) Graph" class="WFChart (엄격한)"("YScale.Maximum"=w80, "YScale.Minimum"=w79, "YScale.ScaleFit"=u8 2 ("Y 스케일.스케일 맞춤")) -> ()  [unwired: 2 in, 2 out]
    }
    frame #2 {
      (unwired) "Init(1)-70lb\t70\t5000\nInit(2)-140lb\t140\t5000\nLoad(1)-0lb\t0\t3000\nLoad(2)-10lb\t10\t3000\nLoad(3)-20lb\t20\t3000\nLoad(4)-40lb\t40\t3000\nLoad(5)-60lb\t60\t3000\nLoad(6)-80lb\t80\t3000"  # 시험용 프로파일 (텍스트)
      w138 = "Init(1)-35lb\t35\t5000\nInit(2)-70lb\t70\t5000\nLoad(1)-0lb\t0\t3000\nLoad(2)-5lb\t5\t3000\nLoad(3)-10lb\t10\t3000\nLoad(4)-20lb\t20\t3000\nLoad(5)-30lb\t30\t3000\nLoad(6)-40lb\t40\t3000"  # 임시 시험용
      # "압력 시험용 프로파일\n(시험명, 인가압력, 시간)"
      # "세로"
      # "Variable initialization"
      n151 = for {
        N: 10 -> [_]
        i -> [w152]
        n152 = Bundle By Name(cluster=T10 {"Row"=0, "Column"=0} ("활성 셀:활성 셀"), "Row"=0, "Column"=w152) -> (w154:T10)
        n153 = property on="Test Data table" class="Tbl (엄격한)"("Active Cell"=w154, "Width"=u32 90 ("활성 셀:셀 크기:폭")) -> ()  [unwired: 2 in, 2 out]
      }
      n154 = for {
        N: 9 -> [_]
        tunnel: [w148] -> w136 mode=indexing
        # "가로"
        n155 = for {
          N: 10 -> [_]
          tunnel: ["-"] -> w148 mode=indexing
        }
      }
      n156 = local write "Mark10 Gauge (lb)"(0.0 ("Mark10 Gauge")) -> ()
      n157 = local write "필터 업데이트"(TRUE ("필터 업데이트")) -> ()
      n158 = local write "FTS 동작시험 상태"(T1 "시험 시작" ("FTS 동작시험 상태")) -> ()
      n159 = local write "FTS comm."(FALSE ("FTS 수신 정상")) -> ()
      n160 = local write "Test name"("Noname" ("Test name")) -> ()
      n161 = local write "FTS Testing"(FALSE ("FTS 시험 진행")) -> ()
      n162 = local write "Test Status"("" ("Force Test Status")) -> ()
      n163 = local write "Load vs Ratio Graph"(cluster{dbl[], dbl[]}[] [] ("Load vs Ratio Graph")) -> ()
      n164 = call "SUB-module-여러줄 문자열을 배열로 변환.vi"("문자열"="Offset (Init)\nOffset (Load)\nInit(1)-70lb\nInit(2)-140lb\nLoad(1)-0lb\nLoad(2)-10lb\nLoad(3)-20lb\nLoad(4)-40lb\nLoad(5)-60lb\nLoad(6)-80lb") -> ("배열"=w133:string[])
      n165 = call "SUB-module-여러줄 문자열을 배열로 변환.vi"("문자열"="Mark10 Gauge(lb)\nLeft Wing-A\nLeft Wing-B\nLeft Wing-C\nLeft Wing-SUM\nRight Wing-A\nRight Wing-B\nRight Wing-C\nRight Wing-SUM") -> ("배열"=w131:string[])
      n166 = local write "Test Data table"(w136) -> ()
      n167 = property on="Test Data table" class="Tbl (엄격한)"("Column Headers[]"=w133) -> ()  [unwired: 2 in, 2 out]
      n168 = property on="Test Data table" class="Tbl (엄격한)"("Row Headers[]"=w131) -> ()  [unwired: 2 in, 2 out]
      n169 = Spreadsheet String To Array(format string="%s" ("포맷 문자열"), spreadsheet string=w138, array type (2D Dbl)=string[][] [] ("배열 타입(2D Dbl)")) -> (array=w141:string[][])  [unwired: 1 in]
      n170 = local write "시험 프로파일"(w141) -> ()
    }
    frame #3 {
      # "프로그램 설정값-파일에서 읽어온다."
      n171 = call "SUB-module-현재 VI 경로.vi"() -> ("현재 VI 경로"=w161:path)
      n172 = Path To String(path=w161) -> (string=w163:string)
      n173 = Concatenate Strings(w163, "\\Configuration File.ini") -> (w162:string)
      n174 = String To Path(string=w162) -> (path=w160:path)
      n175 = call <vilib>:"Open Config Data.vi"("create file if necessary (T)"=TRUE, "configuration file path"=w160) -> ("error out"=w167:errorcluster, "refnum"=w166:T16)  [unwired: 7 in, 1 out]
      n176 = stacked-sequence {
        tunnel: w166 -> [w174 w176 w182]
        tunnel: w167 -> [w173 w175 w181]
        tunnel: "GUI Setting" ("section") -> [w172 w177 _]
        tunnel: [_ _ w182] -> w158
        tunnel: [_ _ w181] -> w157
        frame #0 {
          w171 = "Com Port-Board1"  # Key 1
          n177 = call-poly <vilib>:"Read Key.vi"("section"=w172, "error in (no error)"=w173, "default value"="COM4" ("output string"), "key"=w171, "refnum"=w174) -> ("value"=w170:string)  [unwired: 3 in, 3 out]
          n178 = local write "Port-set 1"(w170) -> ()
        }
        frame #1 {
          w180 = "Com Port-FTS"  # Key 1
          n179 = call-poly <vilib>:"Read Key.vi"("section"=w177, "error in (no error)"=w175, "default value"="COM5" ("output string"), "key"=w180, "refnum"=w176) -> ("value"=w179:string)  [unwired: 3 in, 3 out]
          n180 = local write "Port-FTS"(w179) -> ()
        }
        frame #2 {
        }
      }
      n181 = local write "status string"("Program settings Loading..." ("status string")) -> ()
      n182 = call <vilib>:"Close Config Data.vi"("error in (no error)"=w157, "write file if changed (T)"=FALSE ("write configuration file? (T)"), "refnum"=w158) -> ()  [unwired: 9 out]
    }
    frame #4 {
      n183 = disable-structure shown="비활성화" {
        frame Disabled {
          n184 = while {
            stop <- FALSE stop-if-true
            n185 = Wait Until Next ms Multiple(millisecond multiple=u32 100 ("ms 배수")) -> ()  [unwired: 1 out]
          }
          n186 = local write "Test name"("Noname" ("Test name")) -> ()
          n187 = local write "Test Data table"(string[][] [["0.00", "0.15", "34.85", "70.05", "0.15", "4.90", "9.85", "20.00", "30.10", "39.85"], ["0.99710913", "0.99710572", "0.00000334", "0.00000057", "0.00000226", "-0.00000107", "-0.00000546", "-0.00000098", "-0.00000517", "-0.00001023"], ["0.99966111", "0.99966309", "-0.00000644", "-0.00000672", "-0.00000260", "-0.00000184", "-0.00000479", "-0.00001099", "-0.00001347", "-0.00001280"], ["0.99898257", "0.99898369", "0.00000634", "0.00000730", "0.00000207", "0.00000360", "-0.00000002", "0.00000074", "0.00000350", "0.00000436"], ["-", "-", "0.00000324", "0.00000114", "0.00000174", "0.00000069", "-0.00001028", "-0.00001123", "-0.00001514", "-0.00001867"], ["1.00729492", "1.00730414", "0.00021279", "0.00043786", "0.00000024", "0.00003009", "0.00005593", "0.00011706", "0.00017152", "0.00022235"], ["1.00963793", "1.00965757", "0.00028601", "0.00062313", "-0.00000801", "0.00003538", "0.00007553", "0.00015793", "0.00026760", "0.00037069"], ["1.00040400", "1.00044298", "0.00029371", "0.00059574", "0.00000219", "0.00003805", "0.00007524", "0.00016661", "0.00024595", "0.00031366"], ["-", "-", "0.00079250", "0.00165672", "-0.00000558", "0.00010352", "0.00020671", "0.00044160", "0.00068507", "0.00090671"]] ("Test Data table")) -> ()
        }
        frame Enabled {
        }
      }
      n188 = call "SUB_Delay ms.vi"("delay(ms)"=u32 100 ("ms 타이머 값")) -> ()  [unwired: 3 in]
    }
    frame #5 {
      # "메인 루프"
      n189 = while {
        stop <- w189 stop-if-true
        n190 = stacked-sequence {
          frame #0 {
            # "통신 연결 관리 - RS232"
            n191 = local read "포트닫기 1"() -> (w190:bool)
            n192 = local read "포트오픈 1"() -> (w191:bool)
            n193 = case shown="참" w191 {
              frame False {
              }
              frame True {
                # "통신 연결"
                n194 = stacked-sequence {
                  frame #0 {
                    n195 = local read "Port-set 1"() -> (w196:refnum<visa-resource-name>)
                    n196 = local write "ACT-RS232"(TRUE ("ACT-RS422")) -> ()
                    n197 = local write "데이터 송수신"(TRUE ("Rx")) -> ()
                    n198 = local write "포트오픈 1"(FALSE) -> ()
                    n199 = call "_시리얼 포트-초기화.vi"("baud rate"=u32 115200, "시리얼 포트"=w196) -> ("정상"=w199:bool)  [unwired: 2 in, 1 out]
                    n200 = Wait Until Next ms Multiple(millisecond multiple=u32 500 ("ms 타이머 값")) -> ()  [unwired: 1 out]
                    n201 = local write "Port-act 1"(w196) -> ()
                    n202 = case shown="참" w199 {
                      tunnel: w196 -> [_ w203]
                      frame False {
                        n203 = local write "수신 실패(T) 1"(TRUE ("수신 실패(T) 2")) -> ()
                        n204 = local write "보드-통신상태 1"(FALSE ("Connected")) -> ()
                        n205 = local write "보드 통신 연결 1"(FALSE ("보드 통신 연결 1")) -> ()
                      }
                      frame True {
                        n206 = call "_시리얼-패킷 데이타-수신 - GEN4 1st PP.vi"("ErrIn"=FALSE, "시리얼 포트"=w203) -> ("수신 문자열"=w205:string, "수신 실패(T)"=w204:bool)  [unwired: 2 in, 2 out]
                        n207 = local write "수신 실패(T) 1"(w204) -> ()
                        n208 = case shown="거짓" w204 {
                          tunnel: w205 -> [_ _]
                          frame True {
                            # "수신 데이터 에러 상태"
                            n209 = local read "Port-act 1"() -> (w210:refnum<visa-resource-name>)
                            n210 = VISA Close(VISA resource name=w210) -> ()  [unwired: 1 in, 1 out]
                            n211 = local write "보드-통신상태 1"(FALSE ("Connected")) -> ()
                            n212 = local write "수신 실패(T) 1"(TRUE ("수신 실패(T) 2")) -> ()
                            n213 = local write "*Board ID1"("None...." ("*Board ID")) -> ()
                            n214 = local write "보드 통신 연결 1"(FALSE ("보드 통신 연결 1")) -> ()
                          }
                          frame False {
                            w213 = T2 {"Left Wing-A, C1/C0"=0.0, "Left Wing-B, C2/C0"=0.0, "Left Wing-C, C3/C0"=0.0, "Right Wing-A, C4/C0"=0.0, "Right Wing-B, C5/C0"=0.0, "Right Wing-C, C6/C0"=0.0} ("CDC data")
                            w212 = T4 {"Gyroscope X"=0.0, "Gyroscope Y"=0.0, "Gyroscope Z"=0.0, "Accelerometer X"=0.0, "Accelerometer Y"=0.0, "Accelerometer Z"=0.0} ("IMU data")
                            # "수신 데이터 정상"
                            n215 = local write "CDC Offet"(w213) -> ()
                            n216 = local write "IMU data"(w212) -> ()
                            n217 = local write "IMU Offet"(w212) -> ()
                            n218 = local write "CDC data"(w213) -> ()
                            n219 = Wait Until Next ms Multiple(millisecond multiple=u32 1000 ("ms 타이머 값")) -> ()  [unwired: 1 out]
                            n220 = local write "*Board ID1"("" ("*Board ID")) -> ()
                            n221 = local write "RxD"("Connection. OK....." ("status string")) -> ()
                            n222 = local write "그래프 지우기 1"(TRUE ("그래프 지우기")) -> ()
                            n223 = local write "그래프 지우기 2"(TRUE ("그래프 지우기")) -> ()
                            n224 = local write "통신에러카운트 1"(0 ("통신에러카운트")) -> ()
                            n225 = local write "설정값 로드"(FALSE ("Power On Flag")) -> ()
                            n226 = local write "보드-통신상태 1"(TRUE ("Connected")) -> ()
                            n227 = local write "보드 통신 연결 1"(TRUE ("포트 연결")) -> ()
                          }
                        }
                      }
                    }
                    n228 = local write "status string"("Communication connection attempt.." ("status string")) -> ()
                  }
                  frame #1 {
                    n229 = local write "ACT-RS232"(FALSE ("ACT-RS422")) -> ()
                    n230 = local write "데이터 송수신"(FALSE ("Rx")) -> ()
                  }
                }
              }
            }
            n231 = case shown="참" w190 {
              frame False {
              }
              frame True {
                # "포트 닫기"
                n232 = local write "포트닫기 1"(FALSE ("포트닫기 1")) -> ()
                n233 = local read "Port-act 1"() -> (w231:refnum<visa-resource-name>)
                n234 = local write "status string"("Close communication port." ("status string")) -> ()
                n235 = VISA Close(VISA resource name=w231) -> ()  [unwired: 1 in, 1 out]
                n236 = local write "보드-통신상태 1"(FALSE ("Connected")) -> ()
                n237 = local write "*Board ID1"("None...." ("*Board ID")) -> ()
                n238 = local write "보드 통신 연결 1"(FALSE ("보드 통신 연결 1")) -> ()
                n239 = local write "ACT-RS232"(FALSE ("ACT-RS422")) -> ()
              }
            }
          }
          frame #1 {
            # "모니터링 데이터"
            n240 = local read "보드-통신상태 1"() -> (w232:bool)
            n241 = case shown="참" w232 {
              frame False {
              }
              frame True {
                n242 = stacked-sequence {
                  frame #0 {
                    n243 = local write "수신 실패(T) 1"(FALSE) -> ()
                  }
                  frame #1 {
                    # "데이터 수신"
                    n244 = local read "Port-act 1"() -> (w246:refnum<visa-resource-name>)
                    n245 = local read "수신 실패(T) 1"() -> (w245:bool)
                    n246 = local read "ms 타이머 값"() -> (w240:u32)
                    n247 = Tick Count (ms)() -> (millisecond timer value=w239:u32)
                    n248 = call "_시리얼-패킷 데이타-수신 - GEN4 1st PP.vi"("ErrIn"=w245, "시리얼 포트"=w246) -> ("수신 문자열"=w242:string, "수신 실패(T)"=w243:bool)  [unwired: 2 in, 2 out]
                    n249 = Subtract(x=w239, y=w240) -> (x-y=w237:u32)
                    n250 = local write "status string"("Receive a monitoring data..." ("status string")) -> ()
                    n251 = local write "수신 실패(T) 1"(w243) -> ()
                    n252 = local write "ms 타이머 값"(w239) -> ()
                    n253 = Select(t="Timeout!" ("status string"), s=w243, f=w242) -> (s? t:f=w234:string)
                    n254 = Format Into String(format string="[%d ms] " ("포맷 문자열"), w237) -> (resulting string=w236:string)  [unwired: 2 in, 1 out]
                    n255 = Concatenate Strings(w236, w234) -> (w235:string)
                    n256 = local write "RxD"(w235) -> ()
                  }
                  frame #2 {
                    # "수신 데이터 처리"
                    n257 = local read "수신 실패(T) 1"() -> (w247:bool)
                    n258 = case shown="거짓" w247 {
                      frame False {
                        n259 = stacked-sequence {
                          seq-local: [w248 _ _ _ _ _ _ _] -> [_ w265 w304 _ _ w372 w411 _]
                          seq-local: [w251 _ _ _ _ _ _ _] -> [_ _ _ _ w361 _ _ w415]
                          frame #0 {
                            n260 = local read "그래프 타이머 값 1"() -> (w252:u32)
                            n261 = local read "RxD"() -> (w258:string)
                            n262 = Tick Count (ms)() -> (millisecond timer value=w253:u32)
                            n263 = flat-sequence {
                              tunnel: w253 -> [w263]
                              tunnel: w252 -> [w260]
                              tunnel: [w259] -> w251
                              frame #0 {
                                n264 = Subtract(x=w263, y=w260) -> (x-y=w261:u32)
                                n265 = local write "그래프 타이머 값 1"(w263) -> ()
                                n266 = Multiply(x=w261, y=0.001 ("dt")) -> (x*y=w259:dbl)
                              }
                            }
                            n267 = Match Pattern(string=w258, regular expression="#:" ("검색 문자열"), offset (0)=0 ("오프셋(0)")) -> (after substring=w249:string)  [unwired: 3 out]
                            n268 = Spreadsheet String To Array(delimiter (Tab)="," ("구분 문자(탭)"), format string="%s" ("스프레드시트 문자열"), spreadsheet string=w249, array type (2D Dbl)=string[] [""] ("배열 타입(2D Dbl)")) -> (array=w248:string[])
                            n269 = Array Size(array=w248) -> ()  [unwired: 1 out]
                          }
                          frame #1 {
                            # "펌웨어 버전 (날짜)"
                            n270 = Index Array(array=w265, index=0 ("인덱스")) -> (element=w264:string)
                            n271 = local write "*Board ID1"(w264) -> ()
                          }
                          frame #2 {
                            # "CDC 데이터"
                            n272 = local read "CDC Offet"() -> (w313:T2)
                            n273 = Hexadecimal String To Number(string=w304) -> (number=w274:u32[])  [unwired: 2 in, 1 out]
                            n274 = Unbundle By Name(w313) -> ("Left Wing-A, C1/C0"=w311:dbl, "Left Wing-B, C2/C0"=w305:dbl, "Left Wing-C, C3/C0"=w291:dbl, "Right Wing-A, C4/C0"=w290:dbl, "Right Wing-B, C5/C0"=w289:dbl, "Right Wing-C, C6/C0"=w288:dbl)
                            n275 = Index Array(array=w274, index=1 ("인덱스")) -> (element=w310:u32)
                            n276 = Index Array(array=w274, index=2 ("인덱스")) -> (element=w307:u32)
                            n277 = Index Array(array=w274, index=3 ("인덱스")) -> (element=w299:u32)
                            n278 = Index Array(array=w274, index=4 ("인덱스")) -> (element=w302:u32)
                            n279 = Index Array(array=w274, index=5 ("인덱스")) -> (element=w296:u32)
                            n280 = Index Array(array=w274, index=6 ("인덱스")) -> (element=w293:u32)
                            n281 = call "SUB-자료변환-24Bit 데이터를 실수형(float)으로 변환.vi"("U32"=w310) -> ("FP32"=w309:sgl)  [unwired: 2 in]
                            n282 = call "SUB-자료변환-24Bit 데이터를 실수형(float)으로 변환.vi"("U32"=w307) -> ("FP32"=w308:sgl)  [unwired: 2 in]
                            n283 = call "SUB-자료변환-24Bit 데이터를 실수형(float)으로 변환.vi"("U32"=w299) -> ("FP32"=w300:sgl)  [unwired: 2 in]
                            n284 = call "SUB-자료변환-24Bit 데이터를 실수형(float)으로 변환.vi"("U32"=w302) -> ("FP32"=w301:sgl)  [unwired: 2 in]
                            n285 = call "SUB-자료변환-24Bit 데이터를 실수형(float)으로 변환.vi"("U32"=w296) -> ("FP32"=w295:sgl)  [unwired: 2 in]
                            n286 = call "SUB-자료변환-24Bit 데이터를 실수형(float)으로 변환.vi"("U32"=w293) -> ("FP32"=w294:sgl)  [unwired: 2 in]
                            n287 = Subtract(x=w309, y=w311) -> (x-y=w281:dbl)
                            n288 = Subtract(x=w308, y=w305) -> (x-y=w280:dbl)
                            n289 = Subtract(x=w300, y=w291) -> (x-y=w279:dbl)
                            n290 = Subtract(x=w301, y=w290) -> (x-y=w278:dbl)
                            n291 = Subtract(x=w295, y=w289) -> (x-y=w277:dbl)
                            n292 = Subtract(x=w294, y=w288) -> (x-y=w276:dbl)
                            n293 = Build Array(w281, w280, w279, w278, w277, w276) -> (w284:dbl[])
                            n294 = case shown="거짓" "Filter Enable (CDC)" {
                              tunnel: w284 -> [w314 w316]
                              tunnel: [w314 w315] -> w275
                              frame False {
                                n295 = call "SUB-칼만 필터_CDC.vi"("x set"=w314) -> ()  [unwired: 2 in, 1 out]
                              }
                              frame True {
                                n296 = call "SUB-칼만 필터_CDC.vi"("x set"=w316) -> ("Kalman X"=w315:dbl[])  [unwired: 2 in]
                              }
                            }
                            n297 = In Range and Coerce(upper limit=7.0 ("상위 리미트"), x=w275, lower limit=-7.0 ("하위 리미트")) -> (coerced(x)=w273:dbl[])  [unwired: 1 out]
                            n298 = Index Array(array=w273) -> (element #1=w272:dbl, element #2=w271:dbl, element #3=w270:dbl, element #4=w269:dbl, element #5=w268:dbl, element #6=w267:dbl)  [unwired: 6 in]
                            n299 = local read "CDC data"() -> (w287:T2)
                            n300 = Bundle By Name(cluster=w287, "Left Wing-A, C1/C0"=w272, "Left Wing-B, C2/C0"=w271, "Left Wing-C, C3/C0"=w270, "Right Wing-A, C4/C0"=w269, "Right Wing-B, C5/C0"=w268, "Right Wing-C, C6/C0"=w267) -> (w286:T2)
                            n301 = local write "CDC data"(w286) -> ()
                          }
                          frame #3 {
                            n302 = local read "Fitting Coefficient"() -> (w343:string)
                            n303 = local read "CDC data"() -> (w338:T2)
                            n304 = Unbundle By Name(w338) -> ("Left Wing-A, C1/C0"=w337:dbl, "Left Wing-B, C2/C0"=w336:dbl, "Left Wing-C, C3/C0"=w335:dbl, "Right Wing-A, C4/C0"=w334:dbl, "Right Wing-B, C5/C0"=w333:dbl, "Right Wing-C, C6/C0"=w332:dbl)
                            n305 = Spreadsheet String To Array(format string="%f" ("포맷 문자열"), spreadsheet string=w343) -> (array=w342:dbl[][])  [unwired: 2 in]
                            n306 = Array Subset(array=w342, index (col)=1 ("인덱스")) -> (w340:dbl[][])  [unwired: 3 in]
                            n307 = Array Subset(array=w340, index (row)=1 ("인덱스")) -> (w330:dbl[][])  [unwired: 3 in]
                            n308 = Build Array(w337, w336, w335, w334, w333, w332) -> (w331:dbl[])
                            n309 = Transpose 2D Array(2D array=w330) -> (transposed array=w329:dbl[][])
                            n310 = for {
                              tunnel: w329 -> [w346] mode=indexing
                              tunnel: w331 -> [w347] mode=indexing
                              tunnel: [w345] -> w323 mode=indexing
                              n311 = formula code="float y;\n\ny=cof[0] + x*cof[1]\n      + x*x*cof[2] + x*x*x*cof[3];"("x"=w347, "cof"=w346) -> ("y"=w345:dbl)
                            }
                            n312 = In Range and Coerce(upper limit=9999.0 ("상위 리미트"), x=w323, lower limit=-9999.0 ("하위 리미트")) -> (coerced(x)=w324:dbl[])  [unwired: 1 out]
                            n313 = Index Array(array=w324) -> (element #1=w322:dbl, element #2=w321:dbl, element #3=w320:dbl, element #4=w319:dbl, element #5=w318:dbl, element #6=w317:dbl)  [unwired: 6 in]
                            n314 = local read "CDC data(lb)"() -> (w328:T2)
                            n315 = Bundle By Name(cluster=w328, "Left Wing-A, C1/C0"=w322, "Left Wing-B, C2/C0"=w321, "Left Wing-C, C3/C0"=w320, "Right Wing-A, C4/C0"=w319, "Right Wing-B, C5/C0"=w318, "Right Wing-C, C6/C0"=w317) -> (w327:T2)
                            n316 = local write "CDC data(lb)"(w327) -> ()
                          }
                          frame #4 {
                            # "* 그래프 출력"
                            n317 = local read "CDC data"() -> (w360:T2)
                            n318 = Unbundle By Name(w360) -> ("Left Wing-A, C1/C0"=w359:dbl, "Left Wing-B, C2/C0"=w352:dbl, "Left Wing-C, C3/C0"=w351:dbl, "Right Wing-A, C4/C0"=w350:dbl, "Right Wing-B, C5/C0"=w349:dbl, "Right Wing-C, C6/C0"=w348:dbl)
                            n319 = Build Array(w359) -> (w358:dbl[])
                            n320 = Get Date/Time In Seconds() -> (seconds since 1Jan1904=w364:timestamp)
                            n321 = Build Array(w352) -> (w357:dbl[])
                            n322 = Build Array(w351) -> (w356:dbl[])
                            n323 = Build Array(w349) -> (w354:dbl[])
                            n324 = Build Array(w350) -> (w355:dbl[])
                            n325 = Build Array(w348) -> (w353:dbl[])
                            n326 = Bundle By Name("t0"=w364, "Y"=w358, "dt"=w361) -> (w369:waveform(dbl))  [unwired: 1 in]
                            n327 = Bundle By Name("t0"=w364, "Y"=w357, "dt"=w361) -> (w368:waveform(dbl))  [unwired: 1 in]
                            n328 = Bundle By Name("t0"=w364, "Y"=w356, "dt"=w361) -> (w367:waveform(dbl))  [unwired: 1 in]
                            n329 = Bundle By Name("t0"=w364, "Y"=w355, "dt"=w361) -> (w365:waveform(dbl))  [unwired: 1 in]
                            n330 = Bundle By Name("t0"=w364, "Y"=w354, "dt"=w361) -> (w363:waveform(dbl))  [unwired: 1 in]
                            n331 = Bundle By Name("t0"=w364, "Y"=w353, "dt"=w361) -> (w362:waveform(dbl))  [unwired: 1 in]
                            n332 = Build Array(w369, w368, w367, w365, w363, w362) -> (→"CDC(PCAP02) Graph":waveform(dbl)[])
                          }
                          frame #5 {
                            # "CDC Status"
                            n333 = Hexadecimal String To Number(string=w372) -> (number=w371:u32[])  [unwired: 2 in, 1 out]
                            n334 = Index Array(array=w371, index=7 ("인덱스")) -> (element=→"CDC Status":u32)
                          }
                          frame #6 {
                            n335 = local read "IMU Offet"() -> (w403:T4)
                            n336 = Fract/Exp String To Number(string=w411) -> (number=w404:dbl[])  [unwired: 3 in, 1 out]
                            n337 = local read "Filter Enable (IMU)"() -> (w388:bool)
                            n338 = Unbundle By Name(w403) -> ("Gyroscope X"=w401:dbl, "Gyroscope Y"=w398:dbl, "Gyroscope Z"=w399:dbl, "Accelerometer X"=w394:dbl, "Accelerometer Y"=w393:dbl, "Accelerometer Z"=w392:dbl)
                            n339 = Index Array(array=w404, index=8 ("인덱스")) -> (element=w402:dbl)
                            n340 = Index Array(array=w404, index=9 ("인덱스")) -> (element=w389:dbl)
                            n341 = Index Array(array=w404, index=10 ("인덱스")) -> (element=w400:dbl)
                            n342 = Index Array(array=w404, index=11 ("인덱스")) -> (element=w397:dbl)
                            n343 = Index Array(array=w404, index=12 ("인덱스")) -> (element=w396:dbl)
                            n344 = Index Array(array=w404, index=13 ("인덱스")) -> (element=w395:dbl)
                            n345 = Subtract(x=w402, y=w401) -> (x-y=w385:dbl)
                            n346 = Subtract(x=w389, y=w398) -> (x-y=w384:dbl)
                            n347 = Subtract(x=w400, y=w399) -> (x-y=w383:dbl)
                            n348 = Subtract(x=w397, y=w394) -> (x-y=w382:dbl)
                            n349 = Subtract(x=w396, y=w393) -> (x-y=w381:dbl)
                            n350 = Subtract(x=w395, y=w392) -> (x-y=w380:dbl)
                            n351 = Build Array(w385, w384, w383, w382, w381, w380) -> (w387:dbl[])
                            n352 = case shown="참" w388 {
                              tunnel: w387 -> [w412 w414]
                              tunnel: [w412 w413] -> w386
                              frame False {
                                n353 = call "SUB-칼만 필터_IMU.vi"("x set"=w412) -> ()  [unwired: 2 in, 1 out]
                              }
                              frame True {
                                n354 = call "SUB-칼만 필터_IMU.vi"("x set"=w414) -> ("Kalman X"=w413:dbl[])  [unwired: 2 in]
                              }
                            }
                            n355 = Index Array(array=w386) -> (element #1=w379:dbl, element #2=w378:dbl, element #3=w377:dbl, element #4=w376:dbl, element #5=w375:dbl, element #6=w374:dbl)  [unwired: 6 in]
                            n356 = local read "IMU data"() -> (w391:T4)
                            n357 = Bundle By Name(cluster=w391, "Gyroscope X"=w379, "Gyroscope Y"=w378, "Gyroscope Z"=w377, "Accelerometer X"=w376, "Accelerometer Y"=w375, "Accelerometer Z"=w374) -> (w390:T4)
                            n358 = local write "IMU data"(w390) -> ()
                          }
                          frame #7 {
                            # "* 그래프 출력"
                            n359 = local read "IMU data"() -> (w428:T4)
                            n360 = Unbundle By Name(w428) -> ("Gyroscope X"=w427:dbl, "Gyroscope Y"=w420:dbl, "Gyroscope Z"=w419:dbl, "Accelerometer X"=w418:dbl, "Accelerometer Y"=w417:dbl, "Accelerometer Z"=w416:dbl)
                            n361 = Build Array(w427) -> (w426:dbl[])
                            n362 = Get Date/Time In Seconds() -> (seconds since 1Jan1904=w431:timestamp)
                            n363 = Build Array(w420) -> (w425:dbl[])
                            n364 = Build Array(w419) -> (w424:dbl[])
                            n365 = Build Array(w417) -> (w422:dbl[])
                            n366 = Build Array(w418) -> (w423:dbl[])
                            n367 = Build Array(w416) -> (w421:dbl[])
                            n368 = Bundle By Name("t0"=w431, "Y"=w426, "dt"=w415) -> (w435:waveform(dbl))  [unwired: 1 in]
                            n369 = Bundle By Name("t0"=w431, "Y"=w425, "dt"=w415) -> (w434:waveform(dbl))  [unwired: 1 in]
                            n370 = Bundle By Name("t0"=w431, "Y"=w424, "dt"=w415) -> (w433:waveform(dbl))  [unwired: 1 in]
                            n371 = Bundle By Name("t0"=w431, "Y"=w423, "dt"=w415) -> (w432:waveform(dbl))  [unwired: 1 in]
                            n372 = Bundle By Name("t0"=w431, "Y"=w422, "dt"=w415) -> (w430:waveform(dbl))  [unwired: 1 in]
                            n373 = Bundle By Name("t0"=w431, "Y"=w421, "dt"=w415) -> (w429:waveform(dbl))  [unwired: 1 in]
                            n374 = Build Array(w435, w434, w433, w432, w430, w429) -> (→"IMU Graph":waveform(dbl)[])
                          }
                        }
                      }
                      frame True {
                      }
                    }
                  }
                  frame #3 {
                    n375 = local read "수신 실패(T) 1"() -> (w437:bool)
                    n376 = case shown="거짓" w437 {
                      frame False {
                        # "평균 데이터 취득"
                        n377 = local read "평균데이터 취득-CDC"() -> (w438:bool)
                        n378 = case shown="참" w438 {
                          frame False {
                          }
                          frame True {
                            w445 = 10  # 데이터 수집 횟수
                            n379 = local read "CDC 평균 버퍼"() -> (w449:cluster{"Count":i32, "CDC Data Buffer":T2[]})
                            n380 = local read "CDC data"() -> (w443:T2)
                            n381 = Unbundle By Name(w449) -> ("Count"=w447:i32, "CDC Data Buffer"=w441:T2[])
                            n382 = Build Array(w443) -> (w440:T2[])
                            n383 = Increment(x=w447) -> (x+1=w446:i32)
                            "CDC 평균 카운터" <- w446
                            n384 = Insert Into Array(array=w441, index=0 ("인덱스"), new element=w440) -> (w439:T2[])
                            n385 = Greater Or Equal?(x=w446, y=w445) -> (x >= y?=w444:bool)
                            n386 = case shown="참" w444 {
                              tunnel: w439 -> [_ w467]
                              frame False {
                              }
                              frame True {
                                # "배열 데이터의 평균값을 구하여 치환\n - 평균 버퍼 클리어"
                                n387 = for {
                                tunnel: w467 -> [w474] mode=indexing
                                tunnel: [w473] -> w466 mode=indexing
                                tunnel: [w472] -> w465 mode=indexing
                                tunnel: [w471] -> w464 mode=indexing
                                tunnel: [w470] -> w463 mode=indexing
                                tunnel: [w469] -> w462 mode=indexing
                                tunnel: [w468] -> w461 mode=indexing
                                n388 = Unbundle By Name(w474) -> ("Left Wing-A, C1/C0"=w473:dbl, "Left Wing-B, C2/C0"=w472:dbl, "Left Wing-C, C3/C0"=w471:dbl, "Right Wing-A, C4/C0"=w470:dbl, "Right Wing-B, C5/C0"=w469:dbl, "Right Wing-C, C6/C0"=w468:dbl)
                                }
                                n389 = local write "평균데이터 취득-CDC"(FALSE ("평균데이터 취득-CDC")) -> ()
                                n390 = local write "CDC-평균데이터 처리 완료"(TRUE ("CDC-평균데이터 처리 완료")) -> ()
                                n391 = local write "CDC 평균 버퍼"(cluster{"Count":i32, "CDC Data Buffer":T2[]} {"Count"=0, "CDC Data Buffer"=[]} ("CDC 평균 버퍼")) -> ()
                                n392 = call-poly <vilib>:"Mean.vi"("X"=w466) -> ("mean"=w459:dbl)  [unwired: 1 out]
                                n393 = call-poly <vilib>:"Mean.vi"("X"=w465) -> ("mean"=w458:dbl)  [unwired: 1 out]
                                n394 = call-poly <vilib>:"Mean.vi"("X"=w464) -> ("mean"=w457:dbl)  [unwired: 1 out]
                                n395 = call-poly <vilib>:"Mean.vi"("X"=w463) -> ("mean"=w456:dbl)  [unwired: 1 out]
                                n396 = call-poly <vilib>:"Mean.vi"("X"=w462) -> ("mean"=w455:dbl)  [unwired: 1 out]
                                n397 = call-poly <vilib>:"Mean.vi"("X"=w461) -> ("mean"=w454:dbl)  [unwired: 1 out]
                                n398 = Bundle By Name(cluster=T2 {"Left Wing-A, C1/C0"=0.0, "Left Wing-B, C2/C0"=0.0, "Left Wing-C, C3/C0"=0.0, "Right Wing-A, C4/C0"=0.0, "Right Wing-B, C5/C0"=0.0, "Right Wing-C, C6/C0"=0.0} ("CDC data"), "Left Wing-A, C1/C0"=w459, "Left Wing-B, C2/C0"=w458, "Left Wing-C, C3/C0"=w457, "Right Wing-A, C4/C0"=w456, "Right Wing-B, C5/C0"=w455, "Right Wing-C, C6/C0"=w454) -> (w453:T2)
                                n399 = local write "CDC Averagedata"(w453) -> ()
                              }
                            }
                            n400 = Bundle By Name(cluster=w449, "Count"=w446, "CDC Data Buffer"=w439) -> (w448:cluster{"Count":i32, "CDC Data Buffer":T2[]})
                            n401 = local write "CDC 평균 버퍼"(w448) -> ()
                          }
                        }
                      }
                      frame True {
                      }
                    }
                  }
                  frame #4 {
                    # "데이터 로깅"
                    n402 = local read "수신 실패(T) 1"() -> (w475:bool)
                    n403 = case shown="거짓" w475 {
                      frame False {
                        n404 = local read "Data Logging"() -> (w476:bool)
                        n405 = case shown="참" w476 {
                          frame False {
                            n406 = local read "Logging No."() -> (w478:u32)
                            n407 = Not Equal To 0?(x=w478) -> (x != 0?=w477:bool)
                            n408 = case shown="참" w477 {
                              frame False {
                              }
                              frame True {
                                n409 = local read "log refnum"() -> (w480:refnum<file>)
                                n410 = local write "Logging No."(u32 0 ("Logging No.")) -> ()
                                n411 = Close File(refnum=w480) -> ()  [unwired: 1 in, 2 out]
                              }
                            }
                          }
                          frame True {
                            n412 = stacked-sequence {
                              seq-local: [w481 _] -> [_ w531]
                              frame #0 {
                                n413 = local read "IMU data"() -> (w484:T4)
                                n414 = local read "CDC data"() -> (w501:T2)
                                n415 = Unbundle By Name(w501) -> ("Left Wing-A, C1/C0"=w498:dbl, "Left Wing-B, C2/C0"=w497:dbl, "Left Wing-C, C3/C0"=w496:dbl, "Right Wing-A, C4/C0"=w495:dbl, "Right Wing-B, C5/C0"=w494:dbl, "Right Wing-C, C6/C0"=w493:dbl)
                                n416 = Unbundle By Name(w484) -> ("Gyroscope X"=w487:dbl, "Gyroscope Y"=w488:dbl, "Gyroscope Z"=w489:dbl, "Accelerometer X"=w490:dbl, "Accelerometer Y"=w491:dbl, "Accelerometer Z"=w492:dbl)
                                n417 = Format Into String(format string="%.7f,%.7f,%.7f,%.7f,%.7f,%.7f," ("포맷 문자열"), initial string=",,(GUI) CDC Data," ("포맷 문자열"), w498, w497, w496, w495, w494, w493) -> (resulting string=w483:string)  [unwired: 1 in, 1 out]
                                n418 = Format Into String(format string="%.6f,%.6f,%.6f,%.6f,%.6f,%.6f," ("포맷 문자열"), initial string=",(GUI) IMU Data," ("포맷 문자열"), w487, w488, w489, w490, w491, w492) -> (resulting string=w482:string)  [unwired: 1 in, 1 out]
                                n419 = Concatenate Strings(w483, w482) -> (w481:string)
                              }
                              frame #1 {
                                w525 = T17 1 items=["사용자 홈"=0, "사용자 데스크탑"=1, "사용자 문서"=2, "사용자 어플리케이션 데이터"=3, "사용자 환경"=4, "사용자 임시"=5, "퍼블릭 문서"=6, "퍼블릭 어플리케이션 데이터"=7, "퍼블릭 환경"=8, "퍼블릭 캐시"=13, "시스템 코어 라이브러리"=9, "시스템 설치된 라이브러리"=10, "어플리케이션 파일"=11, "부팅 볼륨 루트"=12] ("system directory type")
                                # "첫행(타이틀)"
                                n420 = local read "Logging No."() -> (w513:u32)
                                n421 = Format Date/Time String(time format string (%c)="Data Logging Start...  %Y/%m/%d %H:%M:%S" ("상태")) -> (date/time string=w504:string)  [unwired: 2 in]
                                n422 = local read "RxD"() -> (w535:string)
                                n423 = call <vilib>:"Get System Directory.vi"("system directory type"=w525) -> ("system directory"=w524:path)  [unwired: 10 in]
                                n424 = Format Into String(format string="\\r\\n\\r\\n%s\\r\\n%s\\r\\n" ("포맷 문자열"), w504, "No.,Time,,Type,F/W ver.,(Raw)Left Wing-A,(Raw)Left Wing-B,(Raw)Left Wing-C,(Raw)Right Wing-A,(Raw)Right Wing-B,(Raw)Right Wing-C,(Raw)CDC Status,(Raw)Gyroscope X,(Raw)Gyroscope Y,(Raw)Gyroscope Z,(Raw)Accelerometer X,(Raw)Accelerometer Y,(Raw)Accelerometer Z,,Type,(GUI)Left Wing-A,(GUI)Left Wing-B,(GUI)Left Wing-C,(GUI)Right Wing-A,(GUI)Right Wing-B,(GUI)Right Wing-C,,Type,(GUI)Gyroscope X,(GUI)Gyroscope Y,(GUI)Gyroscope Z,(GUI)Accelerometer X,(GUI)Accelerometer Y,(GUI)Accelerometer Z" ("문자열")) -> (resulting string=w502:string)  [unwired: 2 in, 1 out]
                                n425 = Increment(x=w513) -> (x+1=w530:u32)
                                n426 = Path To String(path=w524) -> (string=w523:string)
                                n427 = Equal To 0?(x=w513) -> (x = 0?=w511:bool)
                                n428 = Format Date/Time String(time format string (%c)="%Y/%m/%d %H:%M:%S%3u,,RXD Raw Data," ("상태")) -> (date/time string=w537:string)  [unwired: 2 in]
                                n429 = Match Pattern(string=w535, regular expression="#:" ("검색 문자열")) -> (after substring=w533:string)  [unwired: 1 in, 3 out]
                                n430 = Format Into String(format string="%d," ("포맷 문자열"), w513) -> (resulting string=w528:string)  [unwired: 2 in, 1 out]
                                n431 = Concatenate Strings(w523, "\\GEN4 Data Logging.csv" ("문자열")) -> (w521:string)
                                n432 = local write "Logging No."(w530) -> ()
                                n433 = String To Path(string=w521) -> (path=w520:path)
                                n434 = Open/Create/Replace File(file path (use dialog)=w520, operation (0:open)=T11."open or create" ("동작(0:open)"), access (0:read/write)=enum16{"read/write", "read-only", "write-only"}."read/write" ("접근(0:읽기/쓰기)")) -> (refnum out=w515:refnum<file>, error out=w514:errorcluster)  [unwired: 3 in, 1 out]
                                n435 = Select(t=w502, s=w511, f="") -> (s? t:f=w510:string)
                                n436 = Concatenate Strings(w528, w537, w533, w531, "\r\n") -> (w509:string)
                                n437 = Get File Position(4:w514, 7:w515) -> (0:w526:errorcluster, 2:w512:i64, 3:w527:refnum<file>)
                                n438 = Concatenate Strings(w510, w509) -> (w508:string)
                                n439 = call <vilib>:"Write File+ (string).vi"("string"=w508, "error in (no error)"=w526, "pos offset (bytes:0)"=w512, "refnum"=w527) -> ("error out"=w516:errorcluster, "dup refnum"=w517:refnum<file>)  [unwired: 3 in, 1 out]
                                "log refnum" <- w517
                                n440 = disable-structure shown="비활성화" {
                                disable-tunnel: w517 -> [w539 _]
                                disable-tunnel: w516 -> [w538 _]
                                frame Disabled {
                                n441 = Close File(refnum=w539, error in=w538) -> ()  [unwired: 2 out]
                                }
                                frame Enabled {
                                }
                                }
                              }
                            }
                          }
                        }
                      }
                      frame True {
                        n442 = local read "Logging No."() -> (w541:u32)
                        n443 = Not Equal To 0?(x=w541) -> (x != 0?=w540:bool)
                        n444 = case shown="참" w540 {
                          frame False {
                          }
                          frame True {
                            n445 = local read "log refnum"() -> (w543:refnum<file>)
                            n446 = local write "Logging No."(u32 0 ("Logging No.")) -> ()
                            n447 = Close File(refnum=w543) -> ()  [unwired: 1 in, 2 out]
                          }
                        }
                      }
                    }
                  }
                  frame #5 {
                    n448 = local read "수신 실패(T) 1"() -> (w544:bool)
                    n449 = case shown="참" w544 {
                      frame False {
                        n450 = local read "데이터 송수신"() -> (w545:bool)
                        n451 = local read "ACT-RS232"() -> (w546:bool)
                        n452 = Not(x=w546) -> (.not. x?=w547:bool)
                        n453 = Not(x=w545) -> (.not. x?=w548:bool)
                        n454 = local write "데이터 송수신"(w548) -> ()
                        n455 = local write "ACT-RS232"(w547) -> ()
                      }
                      frame True {
                        n456 = local read "통신에러카운트 1"() -> (w551:i32)
                        n457 = Increment(x=w551) -> (x+1=w550:i32)
                        n458 = case shown="10.." w550 {
                          frame 0, Default {
                          }
                          frame 10.. {
                            w552 = FALSE ("포트닫기 1")
                            n459 = local write "포트닫기 1"(TRUE ("포트닫기 1")) -> ()
                            n460 = local write "status string"("Closing the communication port" ("status string")) -> ()
                            n461 = local write "데이터 송수신"(w552) -> ()
                            n462 = local write "ACT-RS232"(w552) -> ()
                            n463 = Wait Until Next ms Multiple(millisecond multiple=u32 1500 ("ms 배수")) -> ()  [unwired: 1 out]
                          }
                        }
                        n464 = local write "통신에러카운트 1"(w550) -> ()
                        n465 = local write "status string"("Communication Error Detected!" ("status string")) -> ()
                      }
                    }
                  }
                }
              }
            }
          }
          frame #2 {
            # "Force Test"
            n466 = local read "수신 실패(T) 1"() -> (w557:bool)
            n467 = local read "Test Start"() -> (w556:bool)
            n468 = case shown="거짓" w557 {
              tunnel: w556 -> [w558 _]
              frame False {
                n469 = case shown="참" w558 {
                  frame False {
                  }
                  frame True {
                    n470 = stacked-sequence {
                      frame #0 {
                        # "세로"
                        # "초기화"
                        n471 = Wait Until Next ms Multiple(millisecond multiple=u32 100 ("ms 배수")) -> ()  [unwired: 1 out]
                        n472 = for {
                          N: 9 -> [_]
                          tunnel: [w570] -> w562 mode=indexing
                          # "가로"
                          n473 = for {
                            N: 10 -> [_]
                            tunnel: ["-"] -> w570 mode=indexing
                          }
                        }
                        n474 = local write "Mark10 Gauge (lb)"(0.0 ("Mark10 Gauge")) -> ()
                        n475 = local write "FTS 동작시험 상태"(T1 "시험 시작" ("FTS 동작시험 상태")) -> ()
                        n476 = local write "FTS Testing"(TRUE ("FTS 시험 진행")) -> ()
                        n477 = local write "FTS comm."(FALSE ("FTS 수신 정상")) -> ()
                        n478 = local write "status string"("Force Test Mode..." ("status string")) -> ()
                        n479 = Format Date/Time String(time format string (%c)="%Y/%m/%d %H:%M:%S> Force Test Start\n" ("상태")) -> (date/time string=w560:string)  [unwired: 2 in]
                        n480 = local write "Test Data table"(w562) -> ()
                        n481 = local write "Test Status"(w560) -> ()
                        n482 = local write "Load vs Ratio Graph"(cluster{dbl[], dbl[]}[] [] ("Load vs Ratio Graph")) -> ()
                      }
                      frame #1 {
                        n483 = local read "Port-FTS"() -> (w578:refnum<visa-resource-name>)
                        n484 = control-ref of="Test Status"() -> (w574:refnum<vi>)
                        n485 = call "_시리얼_Mark10-연결확인.vi"("시리얼 포트"=w578) -> ("수신 정상"=w577:bool, "VISA resource name out"=w576:refnum<visa-resource-name>)  [unwired: 3 in]
                        n486 = call "SUB-Status string update.vi"("텍스트 입력"="Check Serial port of Mark-10\n" ("Force Test Status"), "날짜추가"=TRUE, "reference"=w574) -> ()  [unwired: 2 in, 1 out]
                        n487 = case shown="거짓" w577 {
                          tunnel: w576 -> [_ _]
                          frame False {
                            # "통신 불량"
                            n488 = local write "FTS 동작시험 상태"(T1 "시험 종료" ("FTS 동작시험 상태")) -> ()
                            n489 = One Button Dialog(message="Cannot find MARK10.\nCheck comm port." ("메시지")) -> ()  [unwired: 1 in, 1 out]
                          }
                          frame True {
                          }
                        }
                        n490 = local write "FTS comm."(w577) -> ()
                      }
                      frame #2 {
                        n491 = while {
                          stop <- w584 stop-if-true
                          w581 = FALSE  # 필터 적용
                          # "시험 프로파일"
                          n492 = local read "FTS 동작시험 상태"() -> (w585:T1)
                          n493 = local read "시험 프로파일"() -> (w582:string[][])
                          n494 = Wait Until Next ms Multiple(millisecond multiple=u32 500 ("ms 배수")) -> ()  [unwired: 1 out]
                          n495 = case shown="\"시험 후 점검\"" w585 {
                            tunnel: [w590 _ _ _ _ TRUE] -> w584
                            tunnel: w582 -> [_ _ _ w700 _ _]
                            tunnel: w581 -> [_ _ w595 w699 _ _]
                            frame "시험 시작" {
                              n496 = control-ref of="Test Status"() -> (w587:refnum<vi>)
                              n497 = local write "FTS 동작시험 상태"(T1 "시험전 점검" ("FTS 동작시험 상태")) -> ()
                              n498 = call "SUB-Status string update.vi"("텍스트 입력"="Force Test Start!\n" ("Force Test Status"), "날짜추가"=TRUE, "reference"=w587) -> ()  [unwired: 2 in, 1 out]
                              n499 = local read "stop"() -> (w590:bool)
                            }
                            frame "시험전 점검" {
                              n500 = local read "Port-FTS"() -> (w592:refnum<visa-resource-name>)
                              n501 = call "_시리얼_Mark10-데이터 수신 (게이지).vi"("시리얼 포트"=w592) -> ("데이터(lb)"=w591:dbl, "수신 정상"=w593:bool)  [unwired: 2 in, 1 out]
                              n502 = local write "Mark10 Gauge (lb)"(w591) -> ()
                              n503 = local write "FTS 동작시험 상태"(T1 "시험 진행-CDC 옵셋" ("FTS 동작시험 상태")) -> ()
                              n504 = local write "FTS comm."(w593) -> ()
                            }
                            frame "시험 진행-CDC 옵셋" {
                              n505 = stacked-sequence {
                                tunnel: w595 -> [w596 w612 w641 _ _]
                                frame #0 {
                                # "필터 리셋"
                                n506 = local read "Port-act 1"() -> (w599:refnum<visa-resource-name>)
                                n507 = call "_시리얼-패킷 데이타-수신 - GEN4 1st PP - 전체처리.vi"("CDC Offet"=T2 {"Left Wing-A, C1/C0"=0.0, "Left Wing-B, C2/C0"=0.0, "Left Wing-C, C3/C0"=0.0, "Right Wing-A, C4/C0"=0.0, "Right Wing-B, C5/C0"=0.0, "Right Wing-C, C6/C0"=0.0} ("CDC data"), "필터 적용"=w596, "시리얼 포트"=w599) -> ("CDC data"=w598:T2)  [unwired: 2 in, 2 out]
                                n508 = for {
                                N: 500 -> [_]
                                tunnel: w598 -> [w604]
                                n509 = Unbundle By Name(w604) -> ("Left Wing-A, C1/C0"=w610:dbl, "Left Wing-B, C2/C0"=w609:dbl, "Left Wing-C, C3/C0"=w608:dbl, "Right Wing-A, C4/C0"=w607:dbl, "Right Wing-B, C5/C0"=w606:dbl, "Right Wing-C, C6/C0"=w605:dbl)
                                n510 = Build Array(w610, w609, w608, w607, w606, w605) -> (w611:dbl[])
                                n511 = call "SUB-칼만 필터_CDC.vi"("x set"=w611) -> ()  [unwired: 2 in, 1 out]
                                }
                                n512 = control-ref of="Test Status"() -> (w602:refnum<vi>)
                                n513 = call "SUB-Status string update.vi"("텍스트 입력"="Offset data set... start" ("Force Test Status"), "날짜추가"=TRUE, "reference"=w602) -> ()  [unwired: 2 in, 1 out]
                                }
                                frame #1 {
                                n514 = for {
                                N: 20 -> [_]
                                tunnel: [w637] -> w618 mode=indexing
                                tunnel: [w636] -> w617 mode=indexing
                                tunnel: [w635] -> w616 mode=indexing
                                tunnel: [w634] -> w615 mode=indexing
                                tunnel: [w633] -> w614 mode=indexing
                                tunnel: [w632] -> w613 mode=indexing
                                tunnel: w612 -> [w628]
                                n515 = local read "Port-act 1"() -> (w640:refnum<visa-resource-name>)
                                n516 = local read "Test Status"() -> (w630:string)
                                n517 = call "_시리얼-패킷 데이타-수신 - GEN4 1st PP - 전체처리.vi"("CDC Offet"=T2 {"Left Wing-A, C1/C0"=0.0, "Left Wing-B, C2/C0"=0.0, "Left Wing-C, C3/C0"=0.0, "Right Wing-A, C4/C0"=0.0, "Right Wing-B, C5/C0"=0.0, "Right Wing-C, C6/C0"=0.0} ("CDC data"), "필터 적용"=w628, "시리얼 포트"=w640) -> ("CDC data"=w638:T2)  [unwired: 2 in, 2 out]
                                n518 = Unbundle By Name(w638) -> ("Left Wing-A, C1/C0"=w637:dbl, "Left Wing-B, C2/C0"=w636:dbl, "Left Wing-C, C3/C0"=w635:dbl, "Right Wing-A, C4/C0"=w634:dbl, "Right Wing-B, C5/C0"=w633:dbl, "Right Wing-C, C6/C0"=w632:dbl)
                                n519 = Concatenate Strings(w630, "*") -> (w631:string)
                                n520 = local write "Test Status"(w631) -> ()
                                }
                                n521 = call-poly <vilib>:"Mean.vi"("X"=w618) -> ("mean"=w625:dbl)  [unwired: 1 out]
                                n522 = call-poly <vilib>:"Mean.vi"("X"=w617) -> ("mean"=w624:dbl)  [unwired: 1 out]
                                n523 = call-poly <vilib>:"Mean.vi"("X"=w616) -> ("mean"=w623:dbl)  [unwired: 1 out]
                                n524 = call-poly <vilib>:"Mean.vi"("X"=w615) -> ("mean"=w622:dbl)  [unwired: 1 out]
                                n525 = call-poly <vilib>:"Mean.vi"("X"=w614) -> ("mean"=w621:dbl)  [unwired: 1 out]
                                n526 = call-poly <vilib>:"Mean.vi"("X"=w613) -> ("mean"=w620:dbl)  [unwired: 1 out]
                                n527 = Bundle By Name(cluster=T2 {"Left Wing-A, C1/C0"=0.0, "Left Wing-B, C2/C0"=0.0, "Left Wing-C, C3/C0"=0.0, "Right Wing-A, C4/C0"=0.0, "Right Wing-B, C5/C0"=0.0, "Right Wing-C, C6/C0"=0.0} ("CDC data"), "Left Wing-A, C1/C0"=w625, "Left Wing-B, C2/C0"=w624, "Left Wing-C, C3/C0"=w623, "Right Wing-A, C4/C0"=w622, "Right Wing-B, C5/C0"=w621, "Right Wing-C, C6/C0"=w620) -> (w619:T2)
                                n528 = local write "CDC Offet"(w619) -> ()
                                }
                                frame #2 {
                                n529 = for {
                                N: 20 -> [_]
                                tunnel: [w666] -> w647 mode=indexing
                                tunnel: [w665] -> w646 mode=indexing
                                tunnel: [w664] -> w645 mode=indexing
                                tunnel: [w663] -> w644 mode=indexing
                                tunnel: [w662] -> w643 mode=indexing
                                tunnel: [w661] -> w642 mode=indexing
                                tunnel: w641 -> [w657]
                                n530 = local read "Test Status"() -> (w659:string)
                                n531 = local read "Port-act 1"() -> (w669:refnum<visa-resource-name>)
                                n532 = call "_시리얼-패킷 데이타-수신 - GEN4 1st PP - 전체처리.vi"("CDC Offet"=T2 {"Left Wing-A, C1/C0"=0.0, "Left Wing-B, C2/C0"=0.0, "Left Wing-C, C3/C0"=0.0, "Right Wing-A, C4/C0"=0.0, "Right Wing-B, C5/C0"=0.0, "Right Wing-C, C6/C0"=0.0} ("CDC data"), "필터 적용"=w657, "시리얼 포트"=w669) -> ("CDC data"=w667:T2)  [unwired: 2 in, 2 out]
                                n533 = Concatenate Strings(w659, "#") -> (w660:string)
                                n534 = Unbundle By Name(w667) -> ("Left Wing-A, C1/C0"=w666:dbl, "Left Wing-B, C2/C0"=w665:dbl, "Left Wing-C, C3/C0"=w664:dbl, "Right Wing-A, C4/C0"=w663:dbl, "Right Wing-B, C5/C0"=w662:dbl, "Right Wing-C, C6/C0"=w661:dbl)
                                n535 = local write "Test Status"(w660) -> ()
                                }
                                n536 = call-poly <vilib>:"Mean.vi"("X"=w647) -> ("mean"=w654:dbl)  [unwired: 1 out]
                                n537 = call-poly <vilib>:"Mean.vi"("X"=w646) -> ("mean"=w653:dbl)  [unwired: 1 out]
                                n538 = call-poly <vilib>:"Mean.vi"("X"=w645) -> ("mean"=w652:dbl)  [unwired: 1 out]
                                n539 = call-poly <vilib>:"Mean.vi"("X"=w644) -> ("mean"=w651:dbl)  [unwired: 1 out]
                                n540 = call-poly <vilib>:"Mean.vi"("X"=w643) -> ("mean"=w650:dbl)  [unwired: 1 out]
                                n541 = call-poly <vilib>:"Mean.vi"("X"=w642) -> ("mean"=w649:dbl)  [unwired: 1 out]
                                n542 = Bundle By Name(cluster=T2 {"Left Wing-A, C1/C0"=0.0, "Left Wing-B, C2/C0"=0.0, "Left Wing-C, C3/C0"=0.0, "Right Wing-A, C4/C0"=0.0, "Right Wing-B, C5/C0"=0.0, "Right Wing-C, C6/C0"=0.0} ("CDC data"), "Left Wing-A, C1/C0"=w654, "Left Wing-B, C2/C0"=w653, "Left Wing-C, C3/C0"=w652, "Right Wing-A, C4/C0"=w651, "Right Wing-B, C5/C0"=w650, "Right Wing-C, C6/C0"=w649) -> (w648:T2)
                                n543 = local write "CDC Offet"(w648) -> ()
                                }
                                frame #3 {
                                n544 = local read "Test Status"() -> (w671:string)
                                n545 = Concatenate Strings(w671, "\n") -> (w672:string)
                                n546 = local write "Test Status"(w672) -> ()
                                }
                                frame #4 {
                                w674 = "-"
                                w682 = i16 8 ("정밀도(6)")
                                n547 = local read "CDC Offet"() -> (w695:T2)
                                n548 = control-ref of="Test Status"() -> (w697:refnum<vi>)
                                n549 = Unbundle By Name(w695) -> ("Left Wing-A, C1/C0"=w694:dbl, "Left Wing-B, C2/C0"=w693:dbl, "Left Wing-C, C3/C0"=w692:dbl, "Right Wing-A, C4/C0"=w688:dbl, "Right Wing-B, C5/C0"=w687:dbl, "Right Wing-C, C6/C0"=w686:dbl)
                                n550 = local write "FTS 동작시험 상태"(T1 "시험 진행-압력시험" ("FTS 동작시험 상태")) -> ()
                                n551 = call "SUB-Status string update.vi"("텍스트 입력"="Offset data set... done\n" ("Force Test Status"), "날짜추가"=TRUE, "reference"=w697) -> ()  [unwired: 2 in, 1 out]
                                n552 = local read "Mark10 Gauge (lb)"() -> (w676:dbl)
                                n553 = Number To Fractional String(number=w676, precision (6)=i16 2 ("정밀도(6)")) -> (F-format string=w673:string)  [unwired: 2 in]
                                n554 = Number To Fractional String(number=w694, precision (6)=w682) -> (F-format string=w691:string)  [unwired: 2 in]
                                n555 = Number To Fractional String(number=w693, precision (6)=w682) -> (F-format string=w690:string)  [unwired: 2 in]
                                n556 = Number To Fractional String(number=w692, precision (6)=w682) -> (F-format string=w689:string)  [unwired: 2 in]
                                n557 = Number To Fractional String(number=w688, precision (6)=w682) -> (F-format string=w685:string)  [unwired: 2 in]
                                n558 = Number To Fractional String(number=w687, precision (6)=w682) -> (F-format string=w684:string)  [unwired: 2 in]
                                n559 = Number To Fractional String(number=w686, precision (6)=w682) -> (F-format string=w683:string)  [unwired: 2 in]
                                n560 = local read "Test Data table"() -> (w679:string[][])
                                n561 = Build Array(w673, w691, w690, w689, w674, w685, w684, w683, w674) -> (w681:string[])
                                n562 = Replace Array Subset(array=w679, new element=w681, index (col)=0 ("비활성화된 인덱스 (열)")) -> (w680:string[][])  [unwired: 1 in]
                                n563 = local write "Test Data table"(w680) -> ()
                                }
                              }
                            }
                            frame "시험 진행-압력시험" {
                              n564 = stacked-sequence {
                                tunnel: w700 -> [_ w705 _ _]
                                tunnel: w699 -> [_ w704 _ _]
                                frame #0 {
                                n565 = control-ref of="Test Status"() -> (w702:refnum<vi>)
                                n566 = call "SUB-Status string update.vi"("텍스트 입력"="Start Force test by Profile" ("Force Test Status"), "날짜추가"=TRUE, "reference"=w702) -> ()  [unwired: 2 in, 1 out]
                                }
                                frame #1 {
                                n567 = for {
                                tunnel: w705 -> [w708] mode=indexing
                                tunnel: w704 -> [w706]
                                i -> [w709]
                                stop <- w707 continue-if-true
                                n568 = stacked-sequence {
                                tunnel: w709 -> [w713 _ _ w743 _ w836 w851]
                                tunnel: w708 -> [w712 w725 w730 _ _ _ _]
                                tunnel: [_ w720 _ _ _ _ _] -> w707
                                tunnel: w706 -> [_ _ w727 w742 w793 _ _]
                                frame #0 {
                                # "진행 상태 문자열"
                                n569 = Index Array(array=w712, index=0 ("인덱스")) -> (element=w710:string)
                                n570 = Increment(x=w713) -> (x+1=w714:i32)
                                n571 = control-ref of="Test Status"() -> (w717:refnum<vi>)
                                n572 = Format Into String(format string="Force Testing-Profile(%d)...%s" ("Force Test Status"), w714, w710) -> (resulting string=w716:string)  [unwired: 2 in, 1 out]
                                n573 = call "SUB-Status string update.vi"("텍스트 입력"=w716, "날짜추가"=TRUE, "reference"=w717) -> ()  [unwired: 2 in, 1 out]
                                }
                                frame #1 {
                                # "압력 인가"
                                n574 = Index Array(array=w725, index=1 ("인덱스")) -> (element=w723:string)
                                n575 = local read "Port-FTS"() -> (w726:refnum<visa-resource-name>)
                                n576 = Fract/Exp String To Number(string=w723) -> (number=w722:dbl)  [unwired: 3 in, 1 out]
                                n577 = call "_시리얼_Mark10-제어 (압력설정).vi"("FTS 제어 상태"=T5 "압력제어 시작", "압력 설정(lb)"=w722, "시리얼 포트"=w726) -> ("게이지 압력(lb)"=w719:dbl, "통신 정상"=w720:bool)  [unwired: 1 out]
                                n578 = local write "Mark10 Gauge (lb)"(w719) -> ()
                                n579 = local write "FTS comm."(w720) -> ()
                                }
                                frame #2 {
                                # "대기 시간."
                                n580 = Tick Count (ms)() -> (millisecond timer value=w729:u32)
                                n581 = Index Array(array=w730, index=2 ("인덱스")) -> (element=w731:string)
                                n582 = Fract/Exp String To Number(string=w731) -> (number=w728:dbl)  [unwired: 3 in, 1 out]
                                n583 = while {
                                tunnel: w729 -> [w740]
                                tunnel: w728 -> [w738]
                                tunnel: w727 -> [w733]
                                stop <- w737 stop-if-true
                                n584 = Tick Count (ms)() -> (millisecond timer value=w741:u32)
                                n585 = local read "IMU Offet"() -> (w736:T4)
                                n586 = local read "Port-act 1"() -> (w735:refnum<visa-resource-name>)
                                n587 = Subtract(x=w741, y=w740) -> (x-y=w739:u32)
                                n588 = Greater Or Equal?(x=w739, y=w738) -> (x >= y?=w737:bool)
                                n589 = call "_시리얼-패킷 데이타-수신 - GEN4 1st PP - 전체처리.vi"("CDC Offet"=w736, "필터 적용"=w733, "시리얼 포트"=w735) -> ()  [unwired: 2 in, 3 out]
                                n590 = Wait Until Next ms Multiple(millisecond multiple=u32 20 ("ms 배수")) -> ()  [unwired: 1 out]
                                }
                                }
                                frame #3 {
                                n591 = case shown="2" w743 {
                                tunnel: w742 -> [_ w744]
                                frame 0, Default {
                                }
                                frame 2 {
                                n592 = stacked-sequence {
                                tunnel: w744 -> [w745 _]
                                frame #0 {
                                # "Offset"
                                n593 = for {
                                N: 20 -> [_]
                                tunnel: [w767] -> w751 mode=indexing
                                tunnel: [w766] -> w750 mode=indexing
                                tunnel: [w765] -> w749 mode=indexing
                                tunnel: [w764] -> w748 mode=indexing
                                tunnel: [w763] -> w747 mode=indexing
                                tunnel: [w762] -> w746 mode=indexing
                                tunnel: w745 -> [w761]
                                n594 = local read "Port-act 1"() -> (w770:refnum<visa-resource-name>)
                                n595 = call "_시리얼-패킷 데이타-수신 - GEN4 1st PP - 전체처리.vi"("CDC Offet"=T2 {"Left Wing-A, C1/C0"=0.0, "Left Wing-B, C2/C0"=0.0, "Left Wing-C, C3/C0"=0.0, "Right Wing-A, C4/C0"=0.0, "Right Wing-B, C5/C0"=0.0, "Right Wing-C, C6/C0"=0.0} ("CDC data"), "필터 적용"=w761, "시리얼 포트"=w770) -> ("CDC data"=w768:T2)  [unwired: 2 in, 2 out]
                                n596 = Unbundle By Name(w768) -> ("Left Wing-A, C1/C0"=w767:dbl, "Left Wing-B, C2/C0"=w766:dbl, "Left Wing-C, C3/C0"=w765:dbl, "Right Wing-A, C4/C0"=w764:dbl, "Right Wing-B, C5/C0"=w763:dbl, "Right Wing-C, C6/C0"=w762:dbl)
                                }
                                n597 = call-poly <vilib>:"Mean.vi"("X"=w751) -> ("mean"=w758:dbl)  [unwired: 1 out]
                                n598 = call-poly <vilib>:"Mean.vi"("X"=w750) -> ("mean"=w757:dbl)  [unwired: 1 out]
                                n599 = call-poly <vilib>:"Mean.vi"("X"=w749) -> ("mean"=w756:dbl)  [unwired: 1 out]
                                n600 = call-poly <vilib>:"Mean.vi"("X"=w748) -> ("mean"=w755:dbl)  [unwired: 1 out]
                                n601 = call-poly <vilib>:"Mean.vi"("X"=w747) -> ("mean"=w754:dbl)  [unwired: 1 out]
                                n602 = call-poly <vilib>:"Mean.vi"("X"=w746) -> ("mean"=w753:dbl)  [unwired: 1 out]
                                n603 = Bundle By Name(cluster=T2 {"Left Wing-A, C1/C0"=0.0, "Left Wing-B, C2/C0"=0.0, "Left Wing-C, C3/C0"=0.0, "Right Wing-A, C4/C0"=0.0, "Right Wing-B, C5/C0"=0.0, "Right Wing-C, C6/C0"=0.0} ("CDC data"), "Left Wing-A, C1/C0"=w758, "Left Wing-B, C2/C0"=w757, "Left Wing-C, C3/C0"=w756, "Right Wing-A, C4/C0"=w755, "Right Wing-B, C5/C0"=w754, "Right Wing-C, C6/C0"=w753) -> (w752:T2)
                                n604 = local write "CDC Offet"(w752) -> ()
                                }
                                frame #1 {
                                w772 = "-"
                                w779 = i16 8 ("정밀도(6)")
                                n605 = local read "CDC Offet"() -> (w792:T2)
                                n606 = Unbundle By Name(w792) -> ("Left Wing-A, C1/C0"=w791:dbl, "Left Wing-B, C2/C0"=w790:dbl, "Left Wing-C, C3/C0"=w789:dbl, "Right Wing-A, C4/C0"=w785:dbl, "Right Wing-B, C5/C0"=w784:dbl, "Right Wing-C, C6/C0"=w783:dbl)
                                n607 = local read "Mark10 Gauge (lb)"() -> (w774:dbl)
                                n608 = local read "Test Data table"() -> (w776:string[][])
                                n609 = Number To Fractional String(number=w774, precision (6)=i16 2 ("정밀도(6)")) -> (F-format string=w771:string)  [unwired: 2 in]
                                n610 = Number To Fractional String(number=w791, precision (6)=w779) -> (F-format string=w788:string)  [unwired: 2 in]
                                n611 = Number To Fractional String(number=w790, precision (6)=w779) -> (F-format string=w787:string)  [unwired: 2 in]
                                n612 = Number To Fractional String(number=w789, precision (6)=w779) -> (F-format string=w786:string)  [unwired: 2 in]
                                n613 = Number To Fractional String(number=w785, precision (6)=w779) -> (F-format string=w782:string)  [unwired: 2 in]
                                n614 = Number To Fractional String(number=w784, precision (6)=w779) -> (F-format string=w781:string)  [unwired: 2 in]
                                n615 = Number To Fractional String(number=w783, precision (6)=w779) -> (F-format string=w780:string)  [unwired: 2 in]
                                n616 = Build Array(w771, w788, w787, w786, w772, w782, w781, w780, w772) -> (w778:string[])
                                n617 = Replace Array Subset(array=w776, new element=w778, index (col)=1 ("비활성화된 인덱스 (열)")) -> (w777:string[][])  [unwired: 1 in]
                                n618 = local write "Test Data table"(w777) -> ()
                                }
                                }
                                }
                                }
                                }
                                frame #4 {
                                # "CDC 데이터 수집"
                                n619 = for {
                                N: 5 -> [_]
                                tunnel: [w817] -> w799 mode=indexing
                                tunnel: [w816] -> w798 mode=indexing
                                tunnel: [w815] -> w797 mode=indexing
                                tunnel: [w814] -> w796 mode=indexing
                                tunnel: [w813] -> w795 mode=indexing
                                tunnel: [w812] -> w794 mode=indexing
                                tunnel: w793 -> [w809]
                                n620 = local read "Port-act 1"() -> (w819:refnum<visa-resource-name>)
                                n621 = local read "CDC Offet"() -> (w811:T2)
                                n622 = call "_시리얼-패킷 데이타-수신 - GEN4 1st PP - 전체처리.vi"("CDC Offet"=w811, "필터 적용"=w809, "시리얼 포트"=w819) -> ("CDC data"=w818:T2)  [unwired: 2 in, 2 out]
                                n623 = Unbundle By Name(w818) -> ("Left Wing-A, C1/C0"=w817:dbl, "Left Wing-B, C2/C0"=w816:dbl, "Left Wing-C, C3/C0"=w815:dbl, "Right Wing-A, C4/C0"=w814:dbl, "Right Wing-B, C5/C0"=w813:dbl, "Right Wing-C, C6/C0"=w812:dbl)
                                n624 = Wait Until Next ms Multiple(millisecond multiple=u32 20 ("ms 배수")) -> ()  [unwired: 1 out]
                                }
                                n625 = call-poly <vilib>:"Mean.vi"("X"=w799) -> ("mean"=w806:dbl)  [unwired: 1 out]
                                n626 = call-poly <vilib>:"Mean.vi"("X"=w798) -> ("mean"=w805:dbl)  [unwired: 1 out]
                                n627 = call-poly <vilib>:"Mean.vi"("X"=w797) -> ("mean"=w804:dbl)  [unwired: 1 out]
                                n628 = call-poly <vilib>:"Mean.vi"("X"=w796) -> ("mean"=w803:dbl)  [unwired: 1 out]
                                n629 = call-poly <vilib>:"Mean.vi"("X"=w795) -> ("mean"=w802:dbl)  [unwired: 1 out]
                                n630 = call-poly <vilib>:"Mean.vi"("X"=w794) -> ("mean"=w801:dbl)  [unwired: 1 out]
                                n631 = Bundle By Name(cluster=T2 {"Left Wing-A, C1/C0"=0.0, "Left Wing-B, C2/C0"=0.0, "Left Wing-C, C3/C0"=0.0, "Right Wing-A, C4/C0"=0.0, "Right Wing-B, C5/C0"=0.0, "Right Wing-C, C6/C0"=0.0} ("CDC data"), "Left Wing-A, C1/C0"=w806, "Left Wing-B, C2/C0"=w805, "Left Wing-C, C3/C0"=w804, "Right Wing-A, C4/C0"=w803, "Right Wing-B, C5/C0"=w802, "Right Wing-C, C6/C0"=w801) -> (w800:T2)
                                n632 = local write "CDC data"(w800) -> ()
                                }
                                frame #5 {
                                w832 = i16 8 ("정밀도(6)")
                                n633 = local read "CDC data"() -> (w846:T2)
                                n634 = Unbundle By Name(w846) -> ("Left Wing-A, C1/C0"=w827:dbl, "Left Wing-B, C2/C0"=w828:dbl, "Left Wing-C, C3/C0"=w829:dbl, "Right Wing-A, C4/C0"=w825:dbl, "Right Wing-B, C5/C0"=w824:dbl, "Right Wing-C, C6/C0"=w823:dbl)
                                n635 = local read "Mark10 Gauge (lb)"() -> (w822:dbl)
                                n636 = Compound Arithmetic op=ADD(w829, w828, w827) -> (w830:dbl)
                                n637 = Compound Arithmetic op=ADD(w825, w824, w823) -> (w826:dbl)
                                n638 = Number To Fractional String(number=w827, precision (6)=w832) -> (F-format string=w845:string)  [unwired: 2 in]
                                n639 = Number To Fractional String(number=w828, precision (6)=w832) -> (F-format string=w844:string)  [unwired: 2 in]
                                n640 = Number To Fractional String(number=w822, precision (6)=i16 2 ("정밀도(6)")) -> (F-format string=w820:string)  [unwired: 2 in]
                                n641 = Number To Fractional String(number=w829, precision (6)=w832) -> (F-format string=w843:string)  [unwired: 2 in]
                                n642 = Number To Fractional String(number=w830, precision (6)=w832) -> (F-format string=w833:string)  [unwired: 2 in]
                                n643 = Number To Fractional String(number=w825, precision (6)=w832) -> (F-format string=w842:string)  [unwired: 2 in]
                                n644 = Number To Fractional String(number=w824, precision (6)=w832) -> (F-format string=w841:string)  [unwired: 2 in]
                                n645 = Number To Fractional String(number=w823, precision (6)=w832) -> (F-format string=w840:string)  [unwired: 2 in]
                                n646 = Number To Fractional String(number=w826, precision (6)=w832) -> (F-format string=w831:string)  [unwired: 2 in]
                                n647 = local read "Test Data table"() -> (w837:string[][])
                                n648 = Build Array(w820, w845, w844, w843, w833, w842, w841, w840, w831) -> (w839:string[])
                                n649 = Add(x=2, y=w836) -> (x+y=w834:i32)
                                n650 = Replace Array Subset(array=w837, new element=w839, index (col)=w834) -> (w838:string[][])  [unwired: 1 in]
                                n651 = local write "Test Data table"(w838) -> ()
                                }
                                frame #6 {
                                # "로드 그래프"
                                n652 = local read "Test Data table"() -> (w858:string[][])
                                n653 = Subtract(x=w851, y=1 ("비활성화된 인덱스 (열)")) -> (x-y=w850:i32)
                                n654 = In Range and Coerce(upper limit=9 ("비활성화된 인덱스 (열)"), x=w850, lower limit=1 ("비활성화된 인덱스 (열)")) -> (coerced(x)=w848:i32)  [unwired: 1 out]
                                n655 = Array Subset(array=w858, index (col)=4 ("비활성화된 인덱스 (열)"), length (col)=w848) -> (w853:string[][])  [unwired: 2 in]
                                n656 = Fract/Exp String To Number(string=w853) -> (number=w857:dbl[][])  [unwired: 3 in, 1 out]
                                n657 = for {
                                N: 8 -> [_]
                                tunnel: [w866] -> w856 mode=indexing
                                tunnel: w857 -> [w865]
                                i -> [w863]
                                # "Y"
                                # "X"
                                n658 = Add(x=1, y=w863) -> (x+y=w861:i32)
                                n659 = Index Array(array=w865, index (row)=0 ("비활성화된 인덱스 (열)")) -> (element=w860:dbl[])  [unwired: 1 in]
                                n660 = Index Array(array=w865, index (row)=w861) -> (element=w859:dbl[])  [unwired: 1 in]
                                n661 = Bundle(w860, w859) -> (w866:cluster{dbl[], dbl[]})  [unwired: 1 in]
                                }
                                "Load vs Ratio Graph" <- w856
                                }
                                }
                                }
                                }
                                frame #2 {
                                n662 = local read "Port-FTS"() -> (w869:refnum<visa-resource-name>)
                                n663 = call "_시리얼_Mark10-제어 (압력설정).vi"("FTS 제어 상태"=T5 "헤더 상단 이동", "시리얼 포트"=w869) -> ("게이지 압력(lb)"=w867:dbl, "통신 정상"=w870:bool)  [unwired: 1 in, 1 out]
                                n664 = local write "Mark10 Gauge (lb)"(w867) -> ()
                                n665 = local write "FTS comm."(w870) -> ()
                                }
                                frame #3 {
                                n666 = local write "FTS 동작시험 상태"(T1 "시험 후 점검" ("FTS 동작시험 상태")) -> ()
                                n667 = control-ref of="Test Status"() -> (w872:refnum<vi>)
                                n668 = call "SUB-Status string update.vi"("텍스트 입력"="Done Force test by Profile\n" ("Force Test Status"), "날짜추가"=TRUE, "reference"=w872) -> ()  [unwired: 2 in, 1 out]
                                }
                              }
                            }
                            frame "시험 후 점검" {
                              # "시험 종료 & \n측정 데이터 저장"
                              n669 = stacked-sequence {
                                seq-local: [_ w891 _ _ _] -> [_ _ _ _ w945]
                                seq-local: [_ _ w904 _ _] -> [_ _ _ _ w938]
                                seq-local: [_ _ _ w933 _] -> [_ _ _ _ w937]
                                seq-local: [_ _ _ w932 _] -> [_ _ _ _ w936]
                                seq-local: [w879 _ _ _ _] -> [_ w890 _ _ _]
                                frame #0 {
                                w887 = T17 1 items=["사용자 홈"=0, "사용자 데스크탑"=1, "사용자 문서"=2, "사용자 어플리케이션 데이터"=3, "사용자 환경"=4, "사용자 임시"=5, "퍼블릭 문서"=6, "퍼블릭 어플리케이션 데이터"=7, "퍼블릭 환경"=8, "퍼블릭 캐시"=13, "시스템 코어 라이브러리"=9, "시스템 설치된 라이브러리"=10, "어플리케이션 파일"=11, "부팅 볼륨 루트"=12] ("system directory type")
                                n670 = call <vilib>:"Get System Directory.vi"("system directory type"=w887) -> ("system directory"=w886:path)  [unwired: 10 in]
                                n671 = Path To String(path=w886) -> (string=w885:string)
                                n672 = Concatenate Strings(w885, "\\GEN4-GUI Test data" ("상태")) -> (w879:string)
                                n673 = String To Path(string=w879) -> (path=w883:path)
                                n674 = call <vilib>:"Check if File or Folder Exists.vi"("path"=w883) -> ("error out"=w880:errorcluster, "file or folder exists?"=w882:bool, "dup path"=w881:path)  [unwired: 8 in]
                                n675 = case shown="거짓" w882 {
                                tunnel: w881 -> [w889 _]
                                tunnel: w880 -> [w888 _]
                                frame False {
                                n676 = Create Folder(path (use dialog)=w889, error in=w888) -> ()  [unwired: 1 in, 3 out]
                                }
                                frame True {
                                }
                                }
                                }
                                frame #1 {
                                # "파일 저장 경로"
                                n677 = local read "Test name"() -> (w896:string)
                                n678 = Format Date/Time String(time format string (%c)="%Y%m%d %H%M%S" ("상태")) -> (date/time string=w895:string)  [unwired: 2 in]
                                n679 = Format Into String(format string="\\\\GEN4 Force Test-%s (%s).xlsx" ("상태"), w895, w896) -> (resulting string=w892:string)  [unwired: 2 in, 1 out]
                                n680 = Concatenate Strings(w890, w892) -> (w897:string)
                                n681 = String To Path(string=w897) -> (path=w891:path)
                                }
                                frame #2 {
                                # "remove sum data"
                                # "Fitting"
                                # "Y:인가압력"
                                n682 = local read "Test Data table"() -> (w919:string[][])
                                n683 = Fract/Exp String To Number(string=w919) -> (number=w913:dbl[][])  [unwired: 3 in, 1 out]
                                n684 = Delete From Array(array=w913, length=1 ("길이"), index (row)=4 ("인덱스 (행)")) -> (array with subset deleted=w908:dbl[][])  [unwired: 1 in, 1 out]
                                n685 = Delete From Array(array=w908, length=1 ("길이"), index (row)=7 ("인덱스 (행)")) -> (array with subset deleted=w903:dbl[][])  [unwired: 1 in, 1 out]
                                n686 = Array Subset(array=w903, index (col)=4 ("인덱스")) -> (w918:dbl[][])  [unwired: 3 in]
                                n687 = Array Subset(array=w903, index (row)=1 ("인덱스 (행)"), length (row)=6 ("인덱스 (행)")) -> (w900:dbl[][])  [unwired: 2 in]
                                n688 = Index Array(array=w918, index (row)=0 ("비활성화된 인덱스 (열)")) -> (element=w915:dbl[])  [unwired: 1 in]
                                n689 = Array Subset(array=w918, index (row)=1 ("인덱스")) -> (w916:dbl[][])  [unwired: 3 in]
                                n690 = Index Array(array=w900, index (col)=1 ("인덱스 (행)")) -> (element=w898:dbl[])  [unwired: 1 in]
                                n691 = for {
                                N: 6 -> [_]
                                tunnel: w916 -> [w931]
                                tunnel: w915 -> [w929]
                                tunnel: [w925] -> w907 mode=indexing
                                tunnel: w898 -> [_] mode=indexing
                                i -> [w926]
                                # "Offset"
                                # "X:CDC data"
                                n692 = Index Array(array=w931, index (row)=w926) -> (element=w924:dbl[])  [unwired: 1 in]
                                n693 = Add(x=w924, y=ext 0.0 ("polynomial order")) -> (x+y=w923:ext[])
                                n694 = Divide(x=w929, y=ext 3.0 ("polynomial order")) -> (x/y=w927:ext[])
                                n695 = call <vilib>:"General Polynomial Fit.vi"("Y"=w927, "polynomial order"=3, "X"=w923) -> ("Polynomial Coefficients"=w925:dbl[])  [unwired: 9 in, 3 out]
                                }
                                n696 = Number To Fractional String(number=w907, precision (6)=i16 15 ("정밀도(6)")) -> (F-format string=w905:string[][])  [unwired: 2 in]
                                n697 = Transpose 2D Array(2D array=w905) -> (transposed array=w904:string[][])
                                }
                                frame #3 {
                                # "column header"
                                # "row header"
                                # "Fotting Table - header"
                                n698 = call "SUB-module-여러줄 문자열을 배열로 변환.vi"("문자열"=" Coefficient X^0\nCoefficient X^1\nCoefficient X^2\nCoefficient X^3") -> ("배열"=w933:string[])
                                n699 = call "SUB-module-여러줄 문자열을 배열로 변환.vi"("문자열"="Left Wing-A\nLeft Wing-B\nLeft Wing-C\nRight Wing-A\nRight Wing-B\nRight Wing-C") -> ("배열"=w932:string[])
                                }
                                frame #4 {
                                w942 = 36 items=["xlRangeAutoFormat3DEffects1"=13, "xlRangeAutoFormat3DEffects2"=14, "xlRangeAutoFormatAccounting1"=4, "xlRangeAutoFormatAccounting2"=5, "xlRangeAutoFormatAccounting3"=6, "xlRangeAutoFormatAccounting4"=17, "xlRangeAutoFormatClassic1"=1, "xlRangeAutoFormatClassic2"=2, "xlRangeAutoFormatClassic3"=3, "xlRangeAutoFormatColor1"=7, "xlRangeAutoFormatColor2"=8, "xlRangeAutoFormatColor3"=9, "xlRangeAutoFormatList1"=10, "xlRangeAutoFormatList2"=11, "xlRangeAutoFormatList3"=12, "xlRangeAutoFormatLocalFormat1"=15, "xlRangeAutoFormatLocalFormat2"=16, "xlRangeAutoFormatLocalFormat3"=19, "xlRangeAutoFormatLocalFormat4"=20, "xlRangeAutoFormatReport1"=21, "xlRangeAutoFormatReport2"=22, "xlRangeAutoFormatReport3"=23, "xlRangeAutoFormatReport4"=24, "xlRangeAutoFormatReport5"=25, "xlRangeAutoFormatReport6"=26, "xlRangeAutoFormatReport7"=27, "xlRangeAutoFormatReport8"=28, "xlRangeAutoFormatReport9"=29, "xlRangeAutoFormatReport10"=30, "xlRangeAutoFormatClassicPivotTable"=31, "xlRangeAutoFormatTable1"=32, "xlRangeAutoFormatTable2"=33, "xlRangeAutoFormatTable3"=34, "xlRangeAutoFormatTable4"=35, "xlRangeAutoFormatTable5"=36, "xlRangeAutoFormatTable6"=37, "xlRangeAutoFormatTable7"=38, "xlRangeAutoFormatTable8"=39, "xlRangeAutoFormatTable9"=40, "xlRangeAutoFormatTable10"=41, "xlRangeAutoFormatPTNone"=42, "xlRangeAutoFormatNone"=-4142, "xlRangeAutoFormatSimple"=-4154] ("auto format (none)")
                                w946 = 1 items=["left", "center", "right"] ("horizontal alignment (left)")
                                w961 = 36 items=["xlRangeAutoFormat3DEffects1"=13, "xlRangeAutoFormat3DEffects2"=14, "xlRangeAutoFormatAccounting1"=4, "xlRangeAutoFormatAccounting2"=5, "xlRangeAutoFormatAccounting3"=6, "xlRangeAutoFormatAccounting4"=17, "xlRangeAutoFormatClassic1"=1, "xlRangeAutoFormatClassic2"=2, "xlRangeAutoFormatClassic3"=3, "xlRangeAutoFormatColor1"=7, "xlRangeAutoFormatColor2"=8, "xlRangeAutoFormatColor3"=9, "xlRangeAutoFormatList1"=10, "xlRangeAutoFormatList2"=11, "xlRangeAutoFormatList3"=12, "xlRangeAutoFormatLocalFormat1"=15, "xlRangeAutoFormatLocalFormat2"=16, "xlRangeAutoFormatLocalFormat3"=19, "xlRangeAutoFormatLocalFormat4"=20, "xlRangeAutoFormatReport1"=21, "xlRangeAutoFormatReport2"=22, "xlRangeAutoFormatReport3"=23, "xlRangeAutoFormatReport4"=24, "xlRangeAutoFormatReport5"=25, "xlRangeAutoFormatReport6"=26, "xlRangeAutoFormatReport7"=27, "xlRangeAutoFormatReport8"=28, "xlRangeAutoFormatReport9"=29, "xlRangeAutoFormatReport10"=30, "xlRangeAutoFormatClassicPivotTable"=31, "xlRangeAutoFormatTable1"=32, "xlRangeAutoFormatTable2"=33, "xlRangeAutoFormatTable3"=34, "xlRangeAutoFormatTable4"=35, "xlRangeAutoFormatTable5"=36, "xlRangeAutoFormatTable6"=37, "xlRangeAutoFormatTable7"=38, "xlRangeAutoFormatTable8"=39, "xlRangeAutoFormatTable9"=40, "xlRangeAutoFormatTable10"=41, "xlRangeAutoFormatPTNone"=42, "xlRangeAutoFormatNone"=-4142, "xlRangeAutoFormatSimple"=-4154] ("auto format (none)")
                                w955 = T18 3 items=["B&W", "4 bits", "8 bits", "24 bits"] ("image depth")
                                n700 = property on="Test Data table" class="Tbl (엄격한)"() -> ("Row Headers[]"=w963:string[])  [unwired: 2 in, 2 out]
                                n701 = local read "Test Data table"() -> (w951:string[][])
                                n702 = property on="Test Data table" class="Tbl (엄격한)"() -> ("Column Headers[]"=w962:string[])  [unwired: 2 in, 2 out]
                                n703 = Transpose 2D Array(2D array=w951) -> (transposed array=w960:string[][])
                                n704 = call <vilib>:"New Report.vi"("window state (normal)"=T14."normal", "report type"=T13."Excel") -> ("report out"=w958:refnum<class "NI_report.lvclass">, "error out"=w959:errorcluster)  [unwired: 12 in]
                                n705 = call-poly <vilib>:"Excel Easy Table.vi"("report in"=w958, "auto format (none)"=w961, "text data"=w960, "error in (no error)"=w959, "row headers"=w962, "column headers"=w963) -> ("report out"=w950:refnum<class "NI_report.lvclass">, "error out"=w949:errorcluster)  [unwired: 5 in, 3 out]
                                n706 = control-ref of="Load vs Ratio Graph"() -> (w954:refnum<vi>)
                                n707 = call <vilib>:"Excel Set Cell Alignment.vi"("report in"=w950, "horizontal alignment (left)"=w946, "error in (no error)"=w949) -> ("report out"=w948:refnum<class "NI_report.lvclass">, "error out"=w947:errorcluster)  [unwired: 11 in]
                                n708 = call-dynamic "Append Control Image to Report.vi"("report in"=w948, "image depth"=w955, "ctrl reference"=w954, "description"="Load vs Ratio Graph", "error in (no error)"=w947, "MS Office parameters"=T12 {"position (Excel)"={"row"=13, "column"=1}, "name (Excel)"="", "bookmark (Word)"=""}) -> ("report out"=w944:refnum<class "NI_report.lvclass">, "error out"=w943:errorcluster)  [unwired: 6 in, 2 out]
                                n709 = call-poly <vilib>:"Excel Easy Table.vi"("report in"=w944, "auto format (none)"=w942, "start (0, 0)"=cluster{"row":i32, "column":i32} {"row"=30, "column"=0}, "text data"=w938, "error in (no error)"=w943, "row headers"=w937, "column headers"=w936) -> ("report out"=w941:refnum<class "NI_report.lvclass">, "error out"=w940:errorcluster)  [unwired: 4 in, 3 out]
                                n710 = call-dynamic "Save Report to File.vi"("report in"=w941, "report file path"=w945, "error in (no error)"=w940) -> ()  [unwired: 11 in, 2 out]
                                }
                              }
                              n711 = control-ref of="Test Status"() -> (w877:refnum<vi>)
                              n712 = call "SUB-Status string update.vi"("텍스트 입력"="Result Data Process\n" ("Force Test Status"), "날짜추가"=TRUE, "reference"=w877) -> ()  [unwired: 2 in, 1 out]
                              n713 = local write "FTS 동작시험 상태"(T1 "시험 종료" ("FTS 동작시험 상태")) -> ()
                            }
                            frame "시험 종료", Default {
                              # "시험 종료"
                              n714 = control-ref of="Test Status"() -> (w968:refnum<vi>)
                              n715 = local write "필터 업데이트"(TRUE ("필터 업데이트")) -> ()
                              n716 = local write "그래프 지우기 1"(TRUE ("그래프 지우기")) -> ()
                              n717 = local write "Mark10 Gauge (lb)"(0.0 ("Mark10 Gauge")) -> ()
                              n718 = call "SUB-Status string update.vi"("텍스트 입력"="Test complete." ("Force Test Status"), "날짜추가"=TRUE, "reference"=w968) -> ()  [unwired: 2 in, 1 out]
                              n719 = call <vilib>:"Beep.vi"() -> ()  [unwired: 12 in]
                            }
                          }
                        }
                      }
                      frame #3 {
                        n720 = local write "FTS comm."(FALSE ("FTS 수신 정상")) -> ()
                        n721 = local write "Test Start"(FALSE ("Test Start")) -> ()
                        n722 = local write "FTS Testing"(FALSE ("FTS 시험 진행")) -> ()
                      }
                    }
                  }
                }
              }
              frame True {
                n723 = local write "FTS Testing"(FALSE ("FTS 시험 진행")) -> ()
                n724 = local write "FTS comm."(FALSE ("FTS 수신 정상")) -> ()
                n725 = local write "Test Start"(FALSE ("Test Start")) -> ()
              }
            }
          }
          frame #3 {
            # "설정값 읽기"
            n726 = disable-structure shown="비활성화" {
              frame Disabled {
                n727 = local read "설정값 로드"() -> (w978:bool)
                n728 = local read "보드-통신상태 1"() -> (w977:bool)
                n729 = case shown="참" w978 {
                  tunnel: w977 -> [_ w979]
                  frame False {
                  }
                  frame True {
                    n730 = stacked-sequence {
                      tunnel: w979 -> [_ w981 _ _]
                      frame #0 {
                        n731 = local write "status string"("Loading setting values ..." ("status string")) -> ()
                      }
                      frame #1 {
                        n732 = case shown="참" w981 {
                          frame False {
                          }
                          frame True {
                            # "RS232"
                            n733 = stacked-sequence {
                              frame #0 {
                                n734 = local write "데이터 송수신"(TRUE ("Rx")) -> ()
                                n735 = local write "ACT-RS232"(TRUE ("ACT-RS422")) -> ()
                                n736 = local write "수신 실패(T) 1"(FALSE) -> ()
                              }
                              frame #1 {
                                n737 = call "SUB_Delay ms.vi"("delay(ms)"=u32 100 ("ms 배수")) -> ()  [unwired: 3 in]
                              }
                              frame #2 {
                                n738 = local read "수신 실패(T) 1"() -> (w988:bool)
                                n739 = case shown="참" w988 {
                                frame False {
                                }
                                frame True {
                                n740 = local write "보드-통신상태 1"(FALSE ("Connected")) -> ()
                                }
                                }
                                n741 = local write "데이터 송수신"(FALSE ("Rx")) -> ()
                                n742 = local write "ACT-RS232"(FALSE ("ACT-RS422")) -> ()
                              }
                            }
                          }
                        }
                      }
                      frame #2 {
                      }
                      frame #3 {
                        n743 = local write "설정값 불러오기"(FALSE ("Power On Flag")) -> ()
                        n744 = local write "status string"("Complete call settings." ("status string")) -> ()
                        n745 = local write "설정값 로드"(FALSE ("Power On Flag")) -> ()
                      }
                    }
                  }
                }
              }
              frame Enabled {
              }
            }
          }
          frame #4 {
            # "설정값 저장"
            n746 = disable-structure shown="비활성화" {
              frame Disabled {
                n747 = local read "보드-통신상태 1"() -> (w993:bool)
                n748 = stacked-sequence {
                  tunnel: w993 -> [w994]
                  frame #0 {
                    n749 = case shown="참" w994 {
                      frame False {
                      }
                      frame True {
                        # "RS232"
                        n750 = stacked-sequence {
                          frame #0 {
                            n751 = disable-structure shown="비활성화" {
                              frame Disabled {
                                # "디지털 설정 Setpoint 레벨(0~100%)"
                                n752 = local read item#-1() -> (w996)
                                n753 = Equal?(x=w996, y=T15 "" ("설정값 선택")) -> (x = y?=w997:bool)
                                n754 = case shown="참" w997 {
                                frame False {
                                }
                                frame True {
                                n755 = local read item#-1() -> (w1003)
                                n756 = local write "ACT-RS232"(TRUE ("ACT-RS422")) -> ()
                                n757 = Number To Fractional String(number=w1003, precision (6)=i16 3 ("정밀도(6)")) -> (F-format string=w1001:string)  [unwired: 2 in]
                                n758 = call <vilib>:"Space Constant.vi"() -> ("String"=w1007:string)
                                n759 = local write "status string"("설정값 전송 - 디지털 설정 Setpoint" ("status string")) -> ()
                                n760 = local read "Port-act 1"() -> (w1008:refnum<visa-resource-name>)
                                n761 = Concatenate Strings("SET_DIGSETPOINT" ("전송 문자열"), w1007, w1001) -> (w1005:string)
                                n762 = call "_시리얼 데이타 전송.vi"("전송 문자열"=w1005, "시리얼 포트"=w1008) -> ()  [unwired: 2 out]
                                n763 = local write "데이터 송수신"(TRUE ("Rx")) -> ()
                                n764 = local write item#-1(T15 "" ("설정값 선택")) -> ()
                                }
                                }
                              }
                              frame Enabled {
                              }
                            }
                          }
                          frame #1 {
                            n765 = local read "ACT-RS232"() -> (w1010:bool)
                            n766 = case shown="참" w1010 {
                              frame False {
                              }
                              frame True {
                                n767 = flat-sequence {
                                frame #0 {
                                n768 = call "SUB_Delay ms.vi"("delay(ms)"=u32 100 ("ms 배수")) -> ()  [unwired: 3 in]
                                }
                                frame #1 {
                                n769 = local write "ACT-RS232"(FALSE ("ACT-RS422")) -> ()
                                }
                                }
                              }
                            }
                            n770 = local write "데이터 송수신"(FALSE ("Rx")) -> ()
                          }
                        }
                      }
                    }
                  }
                }
              }
              frame Enabled {
              }
            }
          }
          frame #5 {
            # "지연 시간, 상태값 리셋"
            n771 = local read "필터 업데이트"() -> (w1013:bool)
            n772 = local read "보드-통신상태 1"() -> (w1019:bool)
            n773 = local read "그래프 지우기 1"() -> (w1018:bool)
            n774 = case shown="참" w1013 {
              frame False {
              }
              frame True {
                # "디지털 필터 데이터 업데이트"
                n775 = local read "보드-통신상태 1"() -> (w1021:bool)
                n776 = case shown="참" w1021 {
                  frame False {
                  }
                  frame True {
                    n777 = local read "CDC Offet"() -> (w1023:T2)
                    n778 = local read "Port-act 1"() -> (w1024:refnum<visa-resource-name>)
                    n779 = call "_시리얼-패킷 데이타-수신 - GEN4 1st PP - 전체처리.vi"("CDC Offet"=w1023, "시리얼 포트"=w1024) -> ("CDC data"=w1022:T2)  [unwired: 3 in, 2 out]
                    n780 = for {
                      N: 500 -> [_]
                      tunnel: w1022 -> [w1026]
                      n781 = Unbundle By Name(w1026) -> ("Left Wing-A, C1/C0"=w1032:dbl, "Left Wing-B, C2/C0"=w1031:dbl, "Left Wing-C, C3/C0"=w1030:dbl, "Right Wing-A, C4/C0"=w1029:dbl, "Right Wing-B, C5/C0"=w1028:dbl, "Right Wing-C, C6/C0"=w1027:dbl)
                      n782 = Build Array(w1032, w1031, w1030, w1029, w1028, w1027) -> (w1033:dbl[])
                      n783 = call "SUB-칼만 필터_CDC.vi"("x set"=w1033) -> ()  [unwired: 2 in, 1 out]
                    }
                  }
                }
                n784 = local write "필터 업데이트"(FALSE ("필터 업데이트")) -> ()
              }
            }
            n785 = Not(x=w1019) -> (.not. x?=w1016:bool)
            n786 = case shown="참" w1016 {
              frame False {
              }
              frame True {
                n787 = local write "status string"("Ready (available after the communication connection)" ("status string")) -> ()
              }
            }
            n788 = case shown="참" w1018 {
              frame False {
              }
              frame True {
                n789 = local write "그래프 지우기 1"(FALSE ("그래프 지우기")) -> ()
                n790 = property on="CDC(PCAP02) Graph" class="WFChart (엄격한)"("History Data"=waveform(dbl)[][] [] ("히스토리 데이터")) -> ()  [unwired: 2 in, 2 out]
              }
            }
            n791 = local read "그래프 반출 2"() -> (w1015:bool)
            n792 = local read "그래프 지우기 2"() -> (w1014:bool)
            n793 = local read "그래프 반출 1"() -> (w1017:bool)
            n794 = case shown="참" w1015 {
              frame False {
              }
              frame True {
                n795 = invoke on="IMU Graph" class="WFChart (엄격한)" method="Export Data to Excel"() -> ()  [unwired: 3 in, 3 out]
                n796 = local write "그래프 반출 2"(FALSE ("그래프 반출")) -> ()
              }
            }
            n797 = case shown="참" w1017 {
              frame False {
              }
              frame True {
                n798 = invoke on="CDC(PCAP02) Graph" class="WFChart (엄격한)" method="Export Data to Excel"() -> ()  [unwired: 3 in, 3 out]
                n799 = local write "그래프 반출 1"(FALSE ("그래프 반출")) -> ()
              }
            }
            n800 = case shown="참" w1014 {
              frame False {
              }
              frame True {
                n801 = local write "그래프 지우기 2"(FALSE ("그래프 지우기")) -> ()
                n802 = property on="IMU Graph" class="WFChart (엄격한)"("History Data"=waveform(dbl)[][] [] ("히스토리 데이터")) -> ()  [unwired: 2 in, 2 out]
              }
            }
          }
          frame #6 {
            # "옵셋 설정 (저장)"
            n803 = local read "CDC-평균데이터 처리 완료"() -> (w1042:bool)
            n804 = case shown="참" w1042 {
              frame False {
              }
              frame True {
                n805 = local read "Offset 1"() -> (w1047:bool)
                n806 = case shown="참" w1047 {
                  frame False {
                  }
                  frame True {
                    n807 = local read "CDC Averagedata"() -> (w1049:T2)
                    n808 = for {
                      N: 500 -> [_]
                      w1054 = 0.0 ("원소")
                      n809 = Build Array(w1054, w1054, w1054, w1054, w1054, w1054) -> (w1053:dbl[])
                      n810 = call "SUB-칼만 필터_CDC.vi"("x set"=w1053) -> ()  [unwired: 2 in, 1 out]
                    }
                    n811 = local write "CDC Offet"(w1049) -> ()
                    n812 = local write "그래프 지우기 1"(TRUE ("그래프 지우기")) -> ()
                    n813 = local write "Offset 1"(FALSE ("Offset 1")) -> ()
                    n814 = call "SUB_Delay ms.vi"("delay(ms)"=u32 200) -> ()  [unwired: 3 in]
                  }
                }
              }
            }
            n815 = local read "Offset 2"() -> (w1041:bool)
            n816 = case shown="참" w1041 {
              frame False {
              }
              frame True {
                n817 = local read "IMU data"() -> (w1045:T4)
                n818 = local write "그래프 지우기 2"(TRUE ("그래프 지우기")) -> ()
                n819 = local write "Offset 2"(FALSE ("Offset 1")) -> ()
                n820 = local write "IMU Offet"(w1045) -> ()
                n821 = call "SUB_Delay ms.vi"("delay(ms)"=u32 200) -> ()  [unwired: 3 in]
              }
            }
          }
          frame #7 {
            n822 = local write "CDC-평균데이터 처리 완료"(FALSE ("CDC-평균데이터 처리 완료")) -> ()
          }
          frame #8 {
            # "디버깅 위해 창의 우측 크게 조정"
            # "창크게"
            n823 = local read "창크게"() -> (w1056:bool)
            n824 = case shown="참" w1056 {
              frame False {
              }
              frame True {
                n825 = First Call?() -> (First Call?: T/F=w1058:bool)
                n826 = case shown="참" w1058 {
                  frame False {
                  }
                  frame True {
                    w1075 = 250  # 확장 창 크기
                    n827 = Current VI's Path() -> (path=w1065:path)
                    n828 = Open VI Reference(vi path=w1065) -> (vi reference=w1066:refnum<vi>, error out=w1067:errorcluster)  [unwired: 5 in]
                    n829 = property class="VI"(reference=w1066, error in=w1067) -> (reference out=w1064:refnum<vi>, error out=w1062:errorcluster, "Front Panel.PanelBounds"=w1060:T19)
                    n830 = Unbundle By Name(w1060) -> ("Left"=w1074:i16, "Top"=w1072:i16, "Right"=w1070:i16, "Bottom"=w1071:i16)
                    n831 = expression code="x/2"(w1075) -> (w1069:i32)
                    n832 = Add(x=w1070, y=w1069) -> (x+y=w1068:i32)
                    n833 = Subtract(x=w1074, y=w1069) -> (x-y=w1073:i32)
                    n834 = Bundle By Name(cluster=w1060, "Left"=w1073, "Top"=w1072, "Right"=w1068, "Bottom"=w1071) -> (w1059:T19)
                    n835 = property class="VI"(reference=w1064, error in=w1062, "Front Panel.PanelBounds"=w1059) -> (reference out=w1063:refnum<vi>, error out=w1061:errorcluster)
                    n836 = Close Reference(reference=w1063, error in (no error)=w1061) -> ()  [unwired: 1 out]
                  }
                }
                n837 = local write "창크게"(FALSE ("창크게")) -> ()
              }
            }
          }
        }
        n838 = Wait Until Next ms Multiple(millisecond multiple=u32 30 ("ms 배수")) -> ()  [unwired: 1 out]
        n839 = local read "stop"() -> (w189:bool)
      }
    }
    frame #6 {
      # "시리얼 포트 닫기"
      n840 = local read "보드 통신 연결 1"() -> (w1076:bool)
      n841 = case shown="참" w1076 {
        frame False {
        }
        frame True {
          n842 = local read "Port-act 1"() -> (w1077:refnum<visa-resource-name>)
          n843 = VISA Close(VISA resource name=w1077) -> ()  [unwired: 1 in, 1 out]
        }
      }
    }
    frame #7 {
      # "프로그램 설정값-파일로 저장한다."
      n844 = call <vilib>:"Open Config Data.vi"("configuration file path"=w1082) -> ("error out"=w1085:errorcluster, "refnum"=w1084:T16)  [unwired: 2 in, 7 out]
      n845 = stacked-sequence {
        tunnel: w1084 -> [w1089 w1092 w1097]
        tunnel: w1085 -> [w1088 w1091 w1096]
        tunnel: "GUI Setting" ("section") -> [w1090 w1093 _]
        tunnel: [_ _ w1097] -> w1081
        tunnel: [_ _ w1096] -> w1080
        frame #0 {
          w1087 = "Com Port-Board1"  # Key 1
          n846 = local read "Port-set 1"() -> (w1086:refnum<visa-resource-name>)
          n847 = call-poly <vilib>:"Write Key.vi"("section"=w1090, "error in (no error)"=w1088, "value"=w1086, "key"=w1087, "refnum"=w1089) -> ()  [unwired: 1 in, 6 out]
        }
        frame #1 {
          w1095 = "Com Port-FTS"  # Key 1
          n848 = local read "Port-FTS"() -> (w1094:refnum<visa-resource-name>)
          n849 = call-poly <vilib>:"Write Key.vi"("section"=w1093, "error in (no error)"=w1091, "value"=w1094, "key"=w1095, "refnum"=w1092) -> ()  [unwired: 1 in, 6 out]
        }
        frame #2 {
        }
      }
      n850 = call <vilib>:"Close Config Data.vi"("error in (no error)"=w1080, "refnum"=w1081) -> ()  [unwired: 1 in, 9 out]
      n851 = call "Read and Write Controls to Automatic Config File.vi"("Action"=RWC_Actions."Write", "Control References"=w1078) -> ()  [unwired: 9 in, 1 out]
    }
    frame #8 {
      # "종료"
      n852 = call "SUB-프런트패널 종료.vi"() -> ()  [unwired: 4 in]
    }
  }
